vi "AlgoStim Telemetry Tool.vi"() -> ()   [LabVIEW 2010]
uses:
  Typedef Command List.ctl
  <vilib>/Instr/_visa.llb/VISA Configure Serial Port (Instr).vi
  MICS_ID Global.vi
panel:
  in  "stop":bool
  out "Busy Flag":string="ERROR"
  out "ERROR":bool
  out "SESSION":bool
  out "IDLE":bool
  out "Response":string
  in  "Tab Control":T1(tab)
  out "Error Flag":string="ERROR"
  in  "Clear Error":bool caption="Search for Device"
  out "Error Monitor":errorcluster
  in  "Query Error":bool caption="Search for Device"
  out "Base Station Errors Query":string
  in  "Dongle Reset":bool caption="Search for Device"
  in  "Base Station RF Control":T2={"CCA Mode"=FALSE, "Manual RF CH:"=2, "Base Station CCA Results"=[], "Update CCA"=FALSE, "RSSI Measurement"=0, "Use Averaging?"=TRUE, "400MHz Wakeup"=FALSE, "Listen\nfor\nEmergency"=FALSE} {"RSSI Measurement" items=["External ADC"=0, "Internal ADC"=2]; "Manual RF CH:" min=1 max=10 step=1}
  in  "Search for Device":T3 {"Detected MICS ID's" format="%06x"}
  in  "Session Control":T4={"Open Session"=FALSE, "Close Session"=FALSE, "TARGET MICS ID"=0, "EXID"=16773121, "Company ID"=187, "Calibrate Antenna on \"Open Session\"? "=TRUE} {"Company ID" format="%02x"; "EXID" format="%06x"; "TARGET MICS ID" format="%06x"}
  out "Link Status":T5={"ImplantID"=0, "CompanyID"=0, "RF_Channel"=4, "RX_Mod"=0, "TX_Mod"=0, "TXBlockSize"=15, "RXBlockSize"=15, "BlocksPerPack"=31} {"BlocksPerPack" items=["1"=1, "2"=2, "3"=3, "4"=4, "5"=5, "6"=6, "7"=7, "8"=8, "9"=9, "10"=10, "11"=11, "12"=12, "13"=13, "14"=14, "15"=15, "16"=16, "17"=17, "18"=18, "19"=19, "20"=20, "21"=21, "22"=22, "23"=23, "24"=24, "25"=25, "26"=26, "27"=27, "28"=28, "29"=29, "30"=30, "31"=31]; "RXBlockSize" items=["2"=2, "3"=3, "4"=4, "5"=5, "6"=6, "7"=7, "8"=8, "9"=9, "10"=10, "11"=11, "12"=12, "13"=13, "14"=14, "15"=15, "16"=16, "17"=17, "18"=18, "19"=19, "20"=20, "21"=21, "22"=22, "23"=23, "24"=24, "25"=25, "26"=26, "27"=27, "28"=28, "29"=29, "30"=30, "31"=31]; "TXBlockSize" items=["2"=2, "3"=3, "4"=4, "5"=5, "6"=6, "7"=7, "8"=8, "9"=9, "10"=10, "11"=11, "12"=12, "13"=13, "14"=14, "15"=15, "16"=16, "17"=17, "18"=18, "19"=19, "20"=20, "21"=21, "22"=22, "23"=23, "24"=24, "25"=25, "26"=26, "27"=27, "28"=28, "29"=29, "30"=30, "31"=31]; "TX_Mod" items=["2FSK-FB"=0, "2FSK"=2, "4FSK"=3]; "RX_Mod" items=["2FSK-FB"=0, "2FSK"=8, "4FSK"=12]; "RF_Channel" items=["0", "1", "2", "3", "4", "5", "6", "7", "8", "9"]; "CompanyID" format="%02x"; "ImplantID" format="%06x"}
  out "Link Quality":T6={"MAX_BIT_ERROR"=FALSE, "MAX_RETRIES"=FALSE, "Corrected Blocks"=2650, "CRC Errors"=2650}
  out "Data Status":T7={"TX_BlockCount"=2650, "RX_BlockCount"=2650, "DataErrorCount"=2650}
  out "Status Flags":T8
  in  "Telem Driver":bool caption="Search for Device"
  in  "Parameters":string
  out "Data":string
  out "bChecksum Valid":bool
  out "tChecksum Valid":bool
  out "Response Token":string
  out "Response Code":string
  in  "Command":T9
  in  "CP_DATA IN":u8[](array[numeric])
  out "CP_DATA OUT":u8[](array[numeric])
  in  "Get VBAT Cont":bool
  in  "Get VBAT Single":bool
  out "ADC Counts":dbl
  out "VBAT (Volts)":dbl format="%.3f"
  out "Charging Status":string
  in  "LoadPatProgSlot":u8=1 min=1 max=10 step=1
  in  "LoadPatProgFromDevice":bool caption="Search for Device"
  in  "PulsePW":u16
  in  "PulsePWDn":bool
  in  "PulsePWUp":bool
  in  "Pulse #":u8=1 min=1 max=4 step=1
  in  "PulseAmpl":u16
  in  "PulseAmpDn":bool
  in  "PulseAmpUp":bool
  in  "Freq Index":u8
  in  "ProgAmpls":u16[](array[numeric])
  in  "FreqDn":bool
  in  "FreqUp":bool
  in  "ProgAmpDn":bool
  in  "ProgAmpUp":bool
  in  "StopStimulation":bool caption="Search for Device"
  in  "StartStimulation":bool caption="Search for Device"
  in  "SetPatProgActive":bool caption="Search for Device"
  in  "SendPatProgToDevice":bool caption="Search for Device"
  in  "UpdatePatProgString":bool caption="Search for Device"
  in  "Patient Program String":string
  in  "ResetPatProgToDefaults":bool caption="Search for Device"
  in  "LoadPatProgFromFile":bool caption="Search for Device"
  in  "SavePatProgToFile":bool caption="Search for Device"
  in  "PatStim":T10={"PA"={"Defined"=FALSE, "Amplitudes"=[0, 0, 0, 0, 0, 0, 0, 0, 0, 0, 0, 0, 0, 0, 0, 0, 0, 0, 0, 0, 0, 0, 0, 0, 0, 0], "Pulse Name"="", "Label.Ch"=["ch1", "ch2", "ch3", "ch4", "ch5", "ch6", "ch7", "ch8", "ch9", "ch10", "ch11", "ch12", "ch13", "ch14", "ch15", "ch16", "ch17", "ch18", "ch19", "ch20", "ch21", "ch22", "ch23", "ch24", "ch25", "ch26"], "Amp Low Limit (uA)"=0, "Amp Step (uA)"=0, "Amp Step Index"=0, "PW Low Limit (uS)"=0, "PW High Limit (uS)"=0, "PW Default (uS)"=0}, "Allowed Freq Indexes"=[], "PB"={"Defined"=FALSE, "Amplitudes"=[0, 0, 0, 0, 0, 0, 0, 0, 0, 0, 0, 0, 0, 0, 0, 0, 0, 0, 0, 0, 0, 0, 0, 0, 0, 0], "Pulse Name"="", "Label.Ch"=["ch1", "ch2", "ch3", "ch4", "ch5", "ch6", "ch7", "ch8", "ch9", "ch10", "ch11", "ch12", "ch13", "ch14", "ch15", "ch16", "ch17", "ch18", "ch19", "ch20", "ch21", "ch22", "ch23", "ch24", "ch25", "ch26"], "Amp Low Limit (uA)"=0, "Amp Step (uA)"=0, "Amp Step Index"=0, "PW Low Limit (uS)"=0, "PW High Limit (uS)"=0, "PW Default (uS)"=0}, "PC"={"Defined"=FALSE, "Amplitudes"=[0, 0, 0, 0, 0, 0, 0, 0, 0, 0, 0, 0, 0, 0, 0, 0, 0, 0, 0, 0, 0, 0, 0, 0, 0, 0], "Pulse Name"="", "Label.Ch"=["ch1", "ch2", "ch3", "ch4", "ch5", "ch6", "ch7", "ch8", "ch9", "ch10", "ch11", "ch12", "ch13", "ch14", "ch15", "ch16", "ch17", "ch18", "ch19", "ch20", "ch21", "ch22", "ch23", "ch24", "ch25", "ch26"], "Amp Low Limit (uA)"=0, "Amp Step (uA)"=0, "Amp Step Index"=0, "PW Low Limit (uS)"=0, "PW High Limit (uS)"=0, "PW Default (uS)"=0}, "PD"={"Defined"=FALSE, "Amplitudes"=[0, 0, 0, 0, 0, 0, 0, 0, 0, 0, 0, 0, 0, 0, 0, 0, 0, 0, 0, 0, 0, 0, 0, 0, 0, 0], "Pulse Name"="", "Label.Ch"=["ch1", "ch2", "ch3", "ch4", "ch5", "ch6", "ch7", "ch8", "ch9", "ch10", "ch11", "ch12", "ch13", "ch14", "ch15", "ch16", "ch17", "ch18", "ch19", "ch20", "ch21", "ch22", "ch23", "ch24", "ch25", "ch26"], "Amp Low Limit (uA)"=0, "Amp Step (uA)"=0, "Amp Step Index"=0, "PW Low Limit (uS)"=0, "PW High Limit (uS)"=0, "PW Default (uS)"=0}, "label.freqindex"=[], "Default Freq Index"=0, "Program Name"="", "Program Number"=0, "Program Defined"=FALSE, "Program Disabled"=FALSE} {"Allowed Freq Indexes" format="%02x"}
  in  "Set Attenuator":bool caption="Search for Device"
  in  "Get Attenuator":bool caption="Search for Device"
  in  "Attenuation (dB)":dbl min=0.0 max=31.75 step=0.25 format="%.2g"
  in  "File Path":path
  in  "ZL Mass Read":bool caption="Search for Device"
  out "Get Data Dec":u8
  in  "Register":u16(ring)=1000 items=["---MANUAL ENTRY---"=1000, "REG_NOREG"=0, "REG_RXBUFF_USED"=1, "REG_RXBUFF_BSIZE"=2, "REG_TXBUFF_USED"=3, "REG_TXBUFF_BSIZE"=4, "REG_TXBUFF_MAXPACKSIZE"=5, "REG_MAC_ERRCLR"=6, "REG_MAC_TRAINNUM"=7, "REG_MAC_SYNCMATCH"=8, "REG_MAC_SYNC1"=9, "REG_MAC_SYNC2"=10, "REG_MAC_SYNC3"=11, "REG_MAC_SYNC4"=12, "REG_MAC_SYNC5"=13, "REG_MAC_MAXBERR"=14, "REG_MAC_ECCORR"=15, "REG_MAC_CRCERR"=16, "REG_MAC_BLKCNT1"=17, "REG_MAC_BLKCNT2"=18, "REG_MAC_IMDTRANSID1"=19, "REG_MAC_IMDTRANSID2"=20, "REG_MAC_IMDTRANSID3"=21, "REG_MAC_COMPANYID"=22, "REG_MAC_MODUSER"=23, "REG_MAC_CHANNEL"=25, "REG_MAC_CLEARWDOG"=26, "REG_MAC_CKCORRTHRESH"=27, "REG_HK_TXADDR"=28, "REG_HK_TXDATA"=29, "REG_HK_TXREPLY"=30, "REG_HK_USERDATA"=31, "REG_HK_USERSTATUS"=32, "REG_HK_LASTADDRESS"=33, "REG_HK_MODE"=34, "REG_MAC_STATUSSEQ"=35, "REG_MAC_MAXRETRIES"=36, "REG_MAC_RESENDTIME"=37, "REG_MAC_POWERSAVETIME"=38, "REG_MAC_HEAD_DET"=39, "REG_MAC_CTRL"=41, "REG_MAC_INITCOM"=42, "REG_INTERFACE_MODE"=43, "REG_TXRXBUFF_BOTH"=44, "REG_TXRXBUFF"=45, "REG_IRQ_RAWSTATUS1"=46, "REG_IRQ_ENABLE1"=47, "REG_IRQ_ENABLESET1"=48, "REG_IRQ_ENABLECLEAR1"=49, "REG_IRQ_RAWSTATUS2"=50, "REG_IRQ_ENABLE2"=51, "REG_IRQ_ENABLESET2"=52, "REG_IRQ_ENABLECLEAR2"=53, "REG_IRQ_STATUS1"=54, "REG_IRQ_STATUS2"=55, "REG_IRQ_AUXSTATUS"=56, "REG_TXBUFF_OVERFLOW"=57, "REG_PO0"=58, "REG_P01"=59, "REG_P02"=60, "REG_P03"=61, "REG_GP0"=62, "REG_GPI"=63, "REG_WAKEUP_245IN"=64, "REG_WAKEUP_COMPANYID"=65, "REG_WAKEUP_IMDTRANSID1"=66, "REG_WAKEUP_IMDTRANSID2"=67, "REG_WAKEUP_IMDTRANSID3"=68, "REG_WAKEUP_CHANNEL"=69, "REG_WAKEUP_MODUSER"=70, "REG_WAKEUP_DEVICEMODE"=71, "REG_WAKEUP_WK_RX_CTRL1"=72, "REG_WAKEUP_STACK_ADDR"=73, "REG_WAKEUP_CTRL"=74, "REG_WAKEUP_STROSCRTRIM"=75, "REG_WAKEUP_BIASTRIM"=76, "REG_WAKEUP_ANT245TUNE"=77, "REG_WAKEUP_WK_RX_RTRIMDET"=78, "REG_WAKEUP_WK_RX_RTRIMDEMOD"=79, "REG_WAKEUP_WK_RX_RSSIGAIN"=80, "REG_WAKEUP_LNAFREQ1"=81, "REG_WAKEUP_STACK"=83, "REG_WAKUP_XOSU"=84, "REG_WAKUP_CNTDROPOUT"=85, "REG_WAKEUP_CRCCTRL"=86, "REG_WAKEUP_CRCWORD1"=87, "REG_WAKEUP_CRCWORD2"=88, "REG_WAKEUP_WK_RX_CTRIM"=89, "REG_WAKEUP_VDDATRIM"=90, "REG_WAKEUP_VDDDTRIM"=91, "REG_WAKEUP_TESTIOBUFEN"=92, "REG_WAKEUP_TESTIOCLAMP"=93, "CORE_RESET_ADDRESS"=94, "CHIP_RESET_ADDRESS"=95, "REG_RF_TXGENCTRL"=96, "REG_RF_TXIFCTRL"=97, "REG_RF_TXRF_SEL_CTRL"=98, "REG_RF_TXRFPWRDEFAULTSET"=99, "REG_RF_RSSITRIM"=100, "REG_RF_TXIFOSCTUNE"=101, "REG_RF_TXIFGAINIMB"=102, "REG_RF_TXIFLOCK"=103, "REG_RF_RXRFLNAGAINTRIM"=104, "REG_RF_RXBIASTR"=105, "REG_RF_RXGENCTRL"=106, "REG_RF_RXIFADCDECLEV"=107, "REG_RF_RXIFDETFILTERTUNE"=108, "REG_RF_RXIFFILTERTUNE"=109, "REG_RF_GENENABLES"=110, "REG_RF_SYNTH_CHANNEL"=111, "REG_TX_RAMP_RTRIM"=112, "REG_TX_RAMP_CTRIM"=113, "REG_RF_XO_TRIM"=114, "REG_RF_SYNTH_SET_TRIM"=115, "REG_RF_ADCCTRL"=116, "REG_RF_ADCOUTPUT"=117, "REG_RF_TXIFAMP"=118, "REG_RF_SYNTH_RTRIM"=119, "REG_RF_SYNTH_CTRIM"=120, "REG_RF_SYNTH_CT"=121, "REG_RF_TXMIXER_IOSTRIM_HIGH_IP"=122, "REG_RF_TXMIXER_IOSTRIM_HIGH_IN"=123, "REG_RF_TXMIXER_IOSTRIM_HIGH_QP"=124, "REG_RF_TXMIXER_IOSTRIM_HIGH_QN"=125, "REG_HX_WUADDR"=126, "REG_REVISION"=127, "REG_NOREG_TEST"=128, "REG_DTEST_RXBUFF"=129, "REG_RXBUFF_NEXT_BLOCK"=130, "REG_RXBUFF_FIRST_IN_PACK"=131, "REG_RXBUFF_FIRST_EMPTY"=132, "REG_MAC_BYPASS"=133, "REG_DTEST_TXBUFF"=134, "REG_TXBUFF_NEXT_BLOCK"=135, "REG_TXBUFF_FIRST_IN_PACK"=136, "REG_TXBUFF_FIRST_EMPTY"=137, "REG_DTEST_SEQ"=138, "REG_DTEST_CKCORR"=139, "REG_MAC_TOPSTATE"=140, "REG_DTEST_INTERFACE"=141, "REG_IFACE_TXRX_BYPASS"=142, "REG_MAC_TXRXWAIT"=143, "REG_MAC_TXRFRAMP"=144, "REG_MAC_TRAINWORD"=145, "REG_MAC_TRAINWORD2"=146, "REG_MAC_SETTINGS"=147, "REG_MAC_CALSELECT1"=148, "REG_MAC_CALSELECT2"=149, "REG_MAC_ANTMATCHSEL"=150, "REG_MAC_ANTTUNESEL1"=151, "REG_MAC_ANTTUNESEL2"=152, "REG_MAC_ANTTUNESEL3"=153, "REG_MAC_ANTTUNESTEP"=154, "REG_MAC_WUMODEBURST"=156, "REG_MAC_WUOFFSHORT"=157, "REG_MAC_WUOFFLONG"=158, "REG_MAC_CLKRECCTRL"=159, "REG_HK_MODE_P2"=162, "REG_MAC_ANTTUNERES1"=164, "REG_MAC_ANTTUNERES2"=165, "REG_INTERFACE_MODE_TEST"=171, "REG_TXRXBUFF_BOTH_P2"=172, "REG_TXRXBUFF_P2"=173, "REG_IRQ_RAWSTATUS1_P2"=174, "REG_MAC_TXIFSTATUS1"=176, "REG_MAC_TXIFSTATUS2"=177, "REG_IRQ_RAWSTATUS2_P2"=178, "REG_MAC_TXIFRAMPDELAY"=179, "REG_MAC_TXIFRAMPSLOPE"=180, "REG_MAX_TXIFRAMP"=181, "REG_IRQ_STATUS1_P2"=182, "REG_IRQ_STATUS2_P2"=183, "REG_IRQ_AUXSTATUS_P2"=184, "REG_MAC_UNLOCK"=188, "REG_MAC_TXIFFREQ"=190, "REG_WAKEUP_TESTCTRL1"=192, "REG_WAKEUP_RX_EN_CNT"=193, "REG_WAKEUP_TESTENABLES"=194, "REG_WAKEUP_DTBI_CTRL"=195, "REG_WAKEUP_DTBO_CTRL"=196, "REG_WAKEUP_TESTIOBUFTEST"=197, "REG_WAKEUP_WK_RX_TESTCTRL1"=198, "REG_WAKEUP_WK_RX_TESTCTRL2"=199, "REG_WAKEUP_SENS_SEQUENCE_CTRL"=200, "REG_WAKEUP_LNABIAS"=201, "REG_WAKEUP_DET_TH_TRIM1"=202, "REG_WAKEUP_LNABIAS_NOM1"=203, "REG_WAKEUP_RX_TSHORT_TRIM1"=204, "REG_WAKEUP_LNABIAS_NOM2"=205, "REG_WAKEUP_RX_TLONG_TRIM1"=206, "REG_WAKEUP_LNA_NEGRTRIM_NOM1"=207, "REG_WAKEUP_RX_TBURST_TRIM1"=208, "REG_WAKEUP_RX_LNA_NEGRTRIM_NOM2"=209, "REG_WAKEUP_RX_BB_G_BW_SEL1"=210, "REG_WAKEUP_WK_RX_DET_IOSTRIM1"=212, "REG_WAKEUP_WK_RX_CTRL2"=214, "REG_WAKEUP_WK_RX_RSSIVOSTRIM"=215, "REG_WAKEUP_LNANEGR_EFF"=216, "REG_WAKEUP_XOSU_FAST"=217, "REG_WAKEUP_STROSCPWIDTH1"=218, "REG_WAKEUP_STROSCPERIOD1"=220, "REG_WAKEUP_STROSCPERIOD2"=221, "REG_WAKEUP_WK_RX_LNA_NEGRTRIM1"=222, "REG_RF_TXTESTENABLE"=224, "REG_RF_TXIFTESTMODE"=225, "REG_RF_RXTESTENABLE"=226, "REG_RF_RXIFTESTCTRL1"=227, "REG_RF_RXIFTESTCTRL2"=228, "REG_RF_RXIFTESTCTRL3"=229, "REG_RF_SYNTH_TESTCTRL1"=230, "REG_RF_SYNTH_TESTCTRL2"=231, "REG_RF_SYNTH_TESTCTRL3"=232, "REG_RF_ADCTEST1"=237, "REG_RF_ADCTEST2"=238, "REG_RF_TXMIXER_IOSTRIM_LOW_IP"=240, "REG_RF_TXMIXER_IOSTRIM_LOW_IN"=241, "REG_RF_TXMIXER_ISOTRIM_LOW_QP"=242, "REG_RF_TXMIXER_IOSTRIM_LOW_QN"=243, "REG_RF_SYNTH_KPD"=244, "REG_RF_SYNTH_LOLEV"=245, "REG_RF_TXRFPWRTUNEANTSET"=246, "REG_RF_TXPD_GAIN_CTRL"=247, "REG_RF_SYNTH_STARTUP"=248, "REG_RF_TXRFANTTUNE_TXMODE"=249, "REG_RF_TXRFANTTUNE_RXMODE"=250, "REG_RF_RXRFANTTUNE_TXMODE"=251, "REG_RF_RXRFANTTUNE_RXMODE"=252, "REG_ANTMATCH1"=253, "REG_ANTMATCH2"=254, "REG_REVISION_P2"=255]
  in  "Set Register":bool caption="Search for Device"
  in  "Get Register":bool caption="Search for Device"
  in  "Use Remote?":bool
  out "Get Data":u8 format="%02x"
  in  "Set Data":u8 format="%02x"
  in  "Address":u16 format="%04x"
  in  "Do Calibration":bool caption="Search for Device"
  in  "CAL_WAKEUP_STROBE_OSC":bool
  in  "MICS Channel":i8
  in  "Execute on Remote?(F)":bool
  in  "CAL_TX_IF_OSC":bool
  in  "CAL_FM_DETECT_AND_RX_IF":bool
  in  "CAL_RX_ADC":bool
  in  "CAL_400_MHZ_TX":bool
  in  "CAL_400_MHZ_RX":bool
  in  "CAL_400_MHZ_ANT":bool
  in  "CAL_24MHZ_CRYSTAL_OSC":bool
  in  "Tick Count":u32
  out "error out":errorcluster
  in  "error in (no error)":errorcluster
  in  "VISA Resource Name":refnum<visa-resource-name>="COM14"
  in  "Default MICS Config":T11={"ConfigFlags"=0, "ImplantID"=1048576, "CompanyID"=187, "Normal_Comm"={"RF_Channel"=4, "UserData"=0, "TX_Mod"=0, "RX_Mod"=0, "RX_BlockSize"=15, "BlockPerPack"=31, "TX_BlockSize"=15}, "Emerg_Comm"={"RF_Channel"=4, "UserData"=0, "TX_Mod"=0, "RX_Mod"=0, "TX_BlockSize"=15, "BlockPerPack"=31, "RX_BlockSize"=15}, "ImplantRev"=4, "245TX_PowerCal"=0, "245TX_Power"=10, "CCA_RSSI_Thresholds"={"ch0"=2650, "ch1"=2650, "ch2"=2650, "ch3"=2650, "ch4"=2650, "ch5"=2650, "ch6"=2650, "ch7"=2650, "ch8"=2650, "ch9"=2650}} {"ImplantID" format="%x"; "Normal_Comm"."RF_Channel" items=["0", "1", "2", "3", "4", "5", "6", "7", "8", "9"]; "Normal_Comm"."UserData" items=["0 - 000"=0, "1 - 001"=16, "2 - 010"=32, "3 - 011"=48, "4 - 100"=64, "5 - 101"=80, "6 - 110"=96, "7 - 111"=112]; "Normal_Comm"."TX_Mod" items=["2FSK-FB"=0, "2FSK"=2, "4FSK"=3]; "Normal_Comm"."RX_Mod" items=["2FSK-FB"=0, "2FSK"=8, "4FSK"=12]; "Normal_Comm"."RX_BlockSize" items=["2"=2, "3"=3, "4"=4, "5"=5, "6"=6, "7"=7, "8"=8, "9"=9, "10"=10, "11"=11, "12"=12, "13"=13, "14"=14, "15"=15, "16"=16, "17"=17, "18"=18, "19"=19, "20"=20, "21"=21, "22"=22, "23"=23, "24"=24, "25"=25, "26"=26, "27"=27, "28"=28, "29"=29, "30"=30, "31"=31]; "Normal_Comm"."BlockPerPack" items=["1"=1, "2"=2, "3"=3, "4"=4, "5"=5, "6"=6, "7"=7, "8"=8, "9"=9, "10"=10, "11"=11, "12"=12, "13"=13, "14"=14, "15"=15, "16"=16, "17"=17, "18"=18, "19"=19, "20"=20, "21"=21, "22"=22, "23"=23, "24"=24, "25"=25, "26"=26, "27"=27, "28"=28, "29"=29, "30"=30, "31"=31]; "Normal_Comm"."TX_BlockSize" items=["2"=2, "3"=3, "4"=4, "5"=5, "6"=6, "7"=7, "8"=8, "9"=9, "10"=10, "11"=11, "12"=12, "13"=13, "14"=14, "15"=15, "16"=16, "17"=17, "18"=18, "19"=19, "20"=20, "21"=21, "22"=22, "23"=23, "24"=24, "25"=25, "26"=26, "27"=27, "28"=28, "29"=29, "30"=30, "31"=31]; "Emerg_Comm"."RF_Channel" items=["0", "1", "2", "3", "4", "5", "6", "7", "8", "9"]; "Emerg_Comm"."UserData" items=["0 - 000"=0, "1 - 001"=16, "2 - 010"=32, "3 - 011"=48, "4 - 100"=64, "5 - 101"=80, "6 - 110"=96, "7 - 111"=112]; "Emerg_Comm"."TX_Mod" items=["2FSK-FB"=0, "2FSK"=2, "4FSK"=3]; "Emerg_Comm"."RX_Mod" items=["2FSK-FB"=0, "2FSK"=8, "4FSK"=12]; "Emerg_Comm"."TX_BlockSize" items=["2"=2, "3"=3, "4"=4, "5"=5, "6"=6, "7"=7, "8"=8, "9"=9, "10"=10, "11"=11, "12"=12, "13"=13, "14"=14, "15"=15, "16"=16, "17"=17, "18"=18, "19"=19, "20"=20, "21"=21, "22"=22, "23"=23, "24"=24, "25"=25, "26"=26, "27"=27, "28"=28, "29"=29, "30"=30, "31"=31]; "Emerg_Comm"."BlockPerPack" items=["1"=1, "2"=2, "3"=3, "4"=4, "5"=5, "6"=6, "7"=7, "8"=8, "9"=9, "10"=10, "11"=11, "12"=12, "13"=13, "14"=14, "15"=15, "16"=16, "17"=17, "18"=18, "19"=19, "20"=20, "21"=21, "22"=22, "23"=23, "24"=24, "25"=25, "26"=26, "27"=27, "28"=28, "29"=29, "30"=30, "31"=31]; "Emerg_Comm"."RX_BlockSize" items=["2"=2, "3"=3, "4"=4, "5"=5, "6"=6, "7"=7, "8"=8, "9"=9, "10"=10, "11"=11, "12"=12, "13"=13, "14"=14, "15"=15, "16"=16, "17"=17, "18"=18, "19"=19, "20"=20, "21"=21, "22"=22, "23"=23, "24"=24, "25"=25, "26"=26, "27"=27, "28"=28, "29"=29, "30"=30, "31"=31]; "ImplantRev" items=["ZL70100"=0, "ZL70101"=1, "ZL70102"=4]; "245TX_PowerCal" items=["-29"=-29, "-4"=-4, "-2"=-2, "0"=0, "2"=2, "4"=4, "6"=6, "8"=8, "10"=10, "12"=12, "14"=14, "16"=16, "18"=18, "20"=20, "22"=22, "24"=24, "26"=26, "27"=27]; "245TX_Power" items=["-29"=-29, "-4"=-4, "-2"=-2, "0"=0, "2"=2, "4"=4, "6"=6, "8"=8, "10"=10, "12"=12, "14"=14, "16"=16, "18"=18, "20"=20, "22"=22, "24"=24, "26"=26, "27"=27]}
  # "400MHz\nWakeup"
  # "Auto CCA"
  # "Battery State of Charge"
  # "x .001205 ="
  # "Program Adjust"
  # "Pulse Adjust"
  # "PA"
  # "PB"
  # "PC"
  # "PD"
  # "Pulse D"
  # "Pulse C"
  # "Pulse B"
  # "Pulse A"
  # "ZL REGISTER PEEK AND POKE"
  # "ZL REGISTER MASS READ TO FILE"
  # "Use \"Register\" menu list for named registers,\nor leave it on \"Manual Entry\" and use the \n\"Address\" control to select a register address.\n          (Add 128 (0x80) to P2 addresses)"
  # "Use this function to copy all Zarlink registers to\na text file."
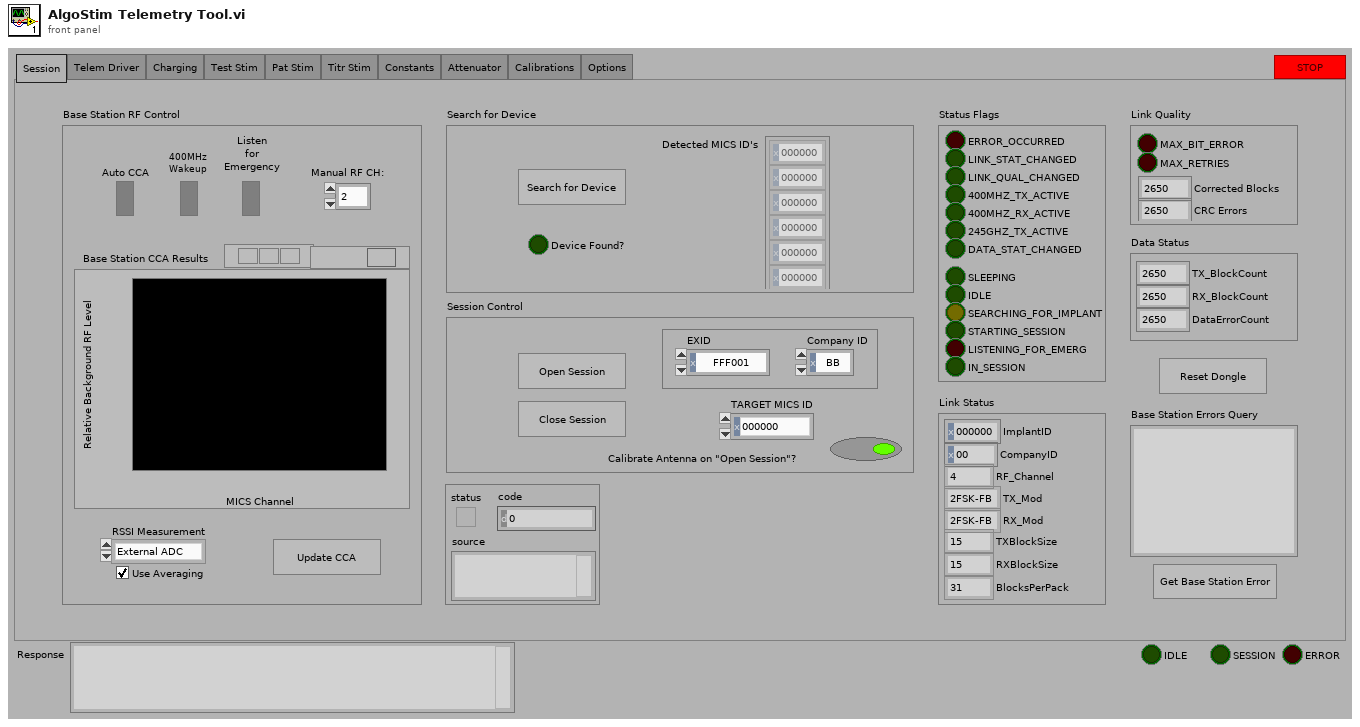
[diagram p1: front panel]
types:
  T1 = enum32{"Session", "Telem Driver", "Charging", "Test Stim", "Pat Stim", "Titr Stim", "Constants", "Attenuator", "Calibrations", "Options"}
  T2 = cluster{"CCA Mode":bool, "Manual RF CH:":u8, "Base Station CCA Results":dbl[], "Update CCA":bool, "RSSI Measurement":u16, "Use Averaging?":bool, "400MHz Wakeup":bool, "Listen\nfor\nEmergency":bool}
  T3 = cluster{"Search for Device":bool, "Device Found?":bool, "Detected MICS ID's":u32[]}
  T4 = cluster{"Open Session":bool, "Close Session":bool, "TARGET MICS ID":u32, "EXID":u32, "Company ID":u8, "Calibrate Antenna on \"Open Session\"? ":bool}
  T5 = cluster{"ImplantID":u32, "CompanyID":u8, "RF_Channel":u8, "RX_Mod":u8, "TX_Mod":u8, "TXBlockSize":u8, "RXBlockSize":u8, "BlocksPerPack":u8}
  T6 = cluster{"MAX_BIT_ERROR":bool, "MAX_RETRIES":bool, "Corrected Blocks":u16, "CRC Errors":u16}
  T7 = cluster{"TX_BlockCount":u16, "RX_BlockCount":u16, "DataErrorCount":u16}
  T8 = cluster{"ERROR_OCCURRED":bool, "LINK_STAT_CHANGED":bool, "LINK_QUAL_CHANGED":bool, "400MHZ_TX_ACTIVE":bool, "400MHZ_RX_ACTIVE":bool, "245GHZ_TX_ACTIVE":bool, "DATA_STAT_CHANGED":bool, "SLEEPING":bool, "IDLE":bool, "SEARCHING_FOR_IMPLANT":bool, "STARTING_SESSION":bool, "LISTENING_FOR_EMERG":bool, "IN_SESSION":bool}
  T9 = typedef "Typedef Command List.ctl" = enum16{"Get xPG Status", "xPG Stimulation", "Select Program", "Increment Program Amplitude", "Decrement Program Amplitude", "Get PoP Constants", "Get PPC Constants", "Get Program Names", "Set Pulse Amplitude", "Increment Pulse Amplitude", "Decrement Pulse Amplitude", "Get Pulse Widths", "Set Pulse Widths", "Increment Pulse Width", "Decrement Pulse Width", "Get Program Frequency", "Set Program Frequency", "Increment Program Frequency", "Decrement Program Frequency", "Inject Event", "Charging Control", "Get xPG Identity", "Set xPG Identity", "Restore Program Defaults", "Get Program Definition", "Set Program Definition", "Get Program Constants", "Set Program Constants", "Get Configurable Device Parameters", "Set Configurable Device Parameters", "Get Pulse Constants", "Set Pulse Constants", "Get Lead Limits", "Set Lead Limits", "Get Channel Calibrations", "Set Channel Calibrations", "<reserved 2>", "<reserved 3>", "<reserved 4>", "<reserved 5>", "<reserved 6>", "<reserved 7>", "Get Stim Asic HV Calibrations", "Set Stim Asic HV Calibrations", "<reserved 8>", "<reserved 9>", "Get CP Data", "Set CP Data", "Clear Log", "Read Log", "Append Log", "Get Patient Program Runtime", "Set Patient Program Runtime", "Impedance Measurement", "Enter Storage Mode", "Echo Short", "Echo Long", "Get General Calibration", "Set General Calibration", "Get Trim List", "Set Trim List", "Get Counter", "Set Counter", "Get Test Stimulation", "Set Test Stimulation", "Get Titration Stimulation", "Set Titration Stimulation", "Get Ramp Time", "Set Ramp Time", "Get VBAT", "Set Software Description Block", "Get Software Description Block", "Write Memory", "Read Memory", "Reset xPG", "Erase Flash Block", "Write Vectors", "Read Vectors", "Diagnostic Data", "Set Background Impedance", "Get Background Impedence ", "Set Test Waveform", "Calibrate Channel", "Get Log Range", "Reserved 0x55", "Reserved 0x56", "MICS Options", "Pair PPC", "Pair POP", "Stop Bootloader", "Tune MICS", "MICS Diagnostics", "Undefined"}
  T10 = cluster{"PA":cluster{"Defined":bool, "Amplitudes":i8[], "Pulse Name":string, "Label.Ch":string[], "Amp Low Limit (uA)":u16, "Amp Step (uA)":u16, "Amp Step Index":u16, "PW Low Limit (uS)":u16, "PW High Limit (uS)":u16, "PW Default (uS)":u16}, "Allowed Freq Indexes":u8[], "PB":cluster{"Defined":bool, "Amplitudes":i8[], "Pulse Name":string, "Label.Ch":string[], "Amp Low Limit (uA)":u16, "Amp Step (uA)":u16, "Amp Step Index":u16, "PW Low Limit (uS)":u16, "PW High Limit (uS)":u16, "PW Default (uS)":u16}, "PC":cluster{"Defined":bool, "Amplitudes":i8[], "Pulse Name":string, "Label.Ch":string[], "Amp Low Limit (uA)":u16, "Amp Step (uA)":u16, "Amp Step Index":u16, "PW Low Limit (uS)":u16, "PW High Limit (uS)":u16, "PW Default (uS)":u16}, "PD":cluster{"Defined":bool, "Amplitudes":i8[], "Pulse Name":string, "Label.Ch":string[], "Amp Low Limit (uA)":u16, "Amp Step (uA)":u16, "Amp Step Index":u16, "PW Low Limit (uS)":u16, "PW High Limit (uS)":u16, "PW Default (uS)":u16}, "label.freqindex":string[], "Default Freq Index":u8, "Program Name":string, "Program Number":u8, "Program Defined":bool, "Program Disabled":bool}
  T11 = cluster{"ConfigFlags":u8, "ImplantID":u32, "CompanyID":u8, "Normal_Comm":cluster{"RF_Channel":u8, "UserData":u8, "TX_Mod":u8, "RX_Mod":u8, "RX_BlockSize":u8, "BlockPerPack":u8, "TX_BlockSize":u8}, "Emerg_Comm":cluster{"RF_Channel":u8, "UserData":u8, "TX_Mod":u8, "RX_Mod":u8, "TX_BlockSize":u8, "BlockPerPack":u8, "RX_BlockSize":u8}, "ImplantRev":u8, "245TX_PowerCal":i8, "245TX_Power":i8, "CCA_RSSI_Thresholds":cluster{"ch0":u16, "ch1":u16, "ch2":u16, "ch3":u16, "ch4":u16, "ch5":u16, "ch6":u16, "ch7":u16, "ch8":u16, "ch9":u16}}
  T12 = cluster{"Command":T9, "Function":enum16{"Open Session", "Close Session", "Downlink Only", "Uplink Only", "Transceive (DN -> UP)"}, "MICS_ID":u32, "EXID":u32, "Use Local":bool, "Transceive Delay mS":dbl, "CP_DATA IN":u8[], "Parameters":string}
  T13 = enum16{"Open Session", "Close Session", "Downlink Only", "Uplink Only", "Transceive (DN -> UP)"}
  T14 = enum16{"Get Device Type", "Get Device Name", "Get Device Version", "Get Device Error"}
  T15 = enum16{"open", "replace", "create", "open or create", "replace or create", "replace or create with confirmation"}
  T16 = cluster{"Response Token":string, "Response Code":string, "bChecksum Valid":bool, "tChecksum Valid":bool, "CP_DATA OUT":u8[], "Data":string}
  T17 = cluster{"Open Session":bool, "Close Session":bool, "TARGET MICS ID":u32, "EXID":u32, "Company ID":u8, bool}
  T18 = cluster{"Allowed Freq Indexes[0]":u8, "Allowed Freq Indexes[1]":u8, "Allowed Freq Indexes[2]":u8, "Allowed Freq Indexes[3]":u8, "Allowed Freq Indexes[4]":u8, "Allowed Freq Indexes[5]":u8, "Allowed Freq Indexes[6]":u8, "Allowed Freq Indexes[7]":u8}
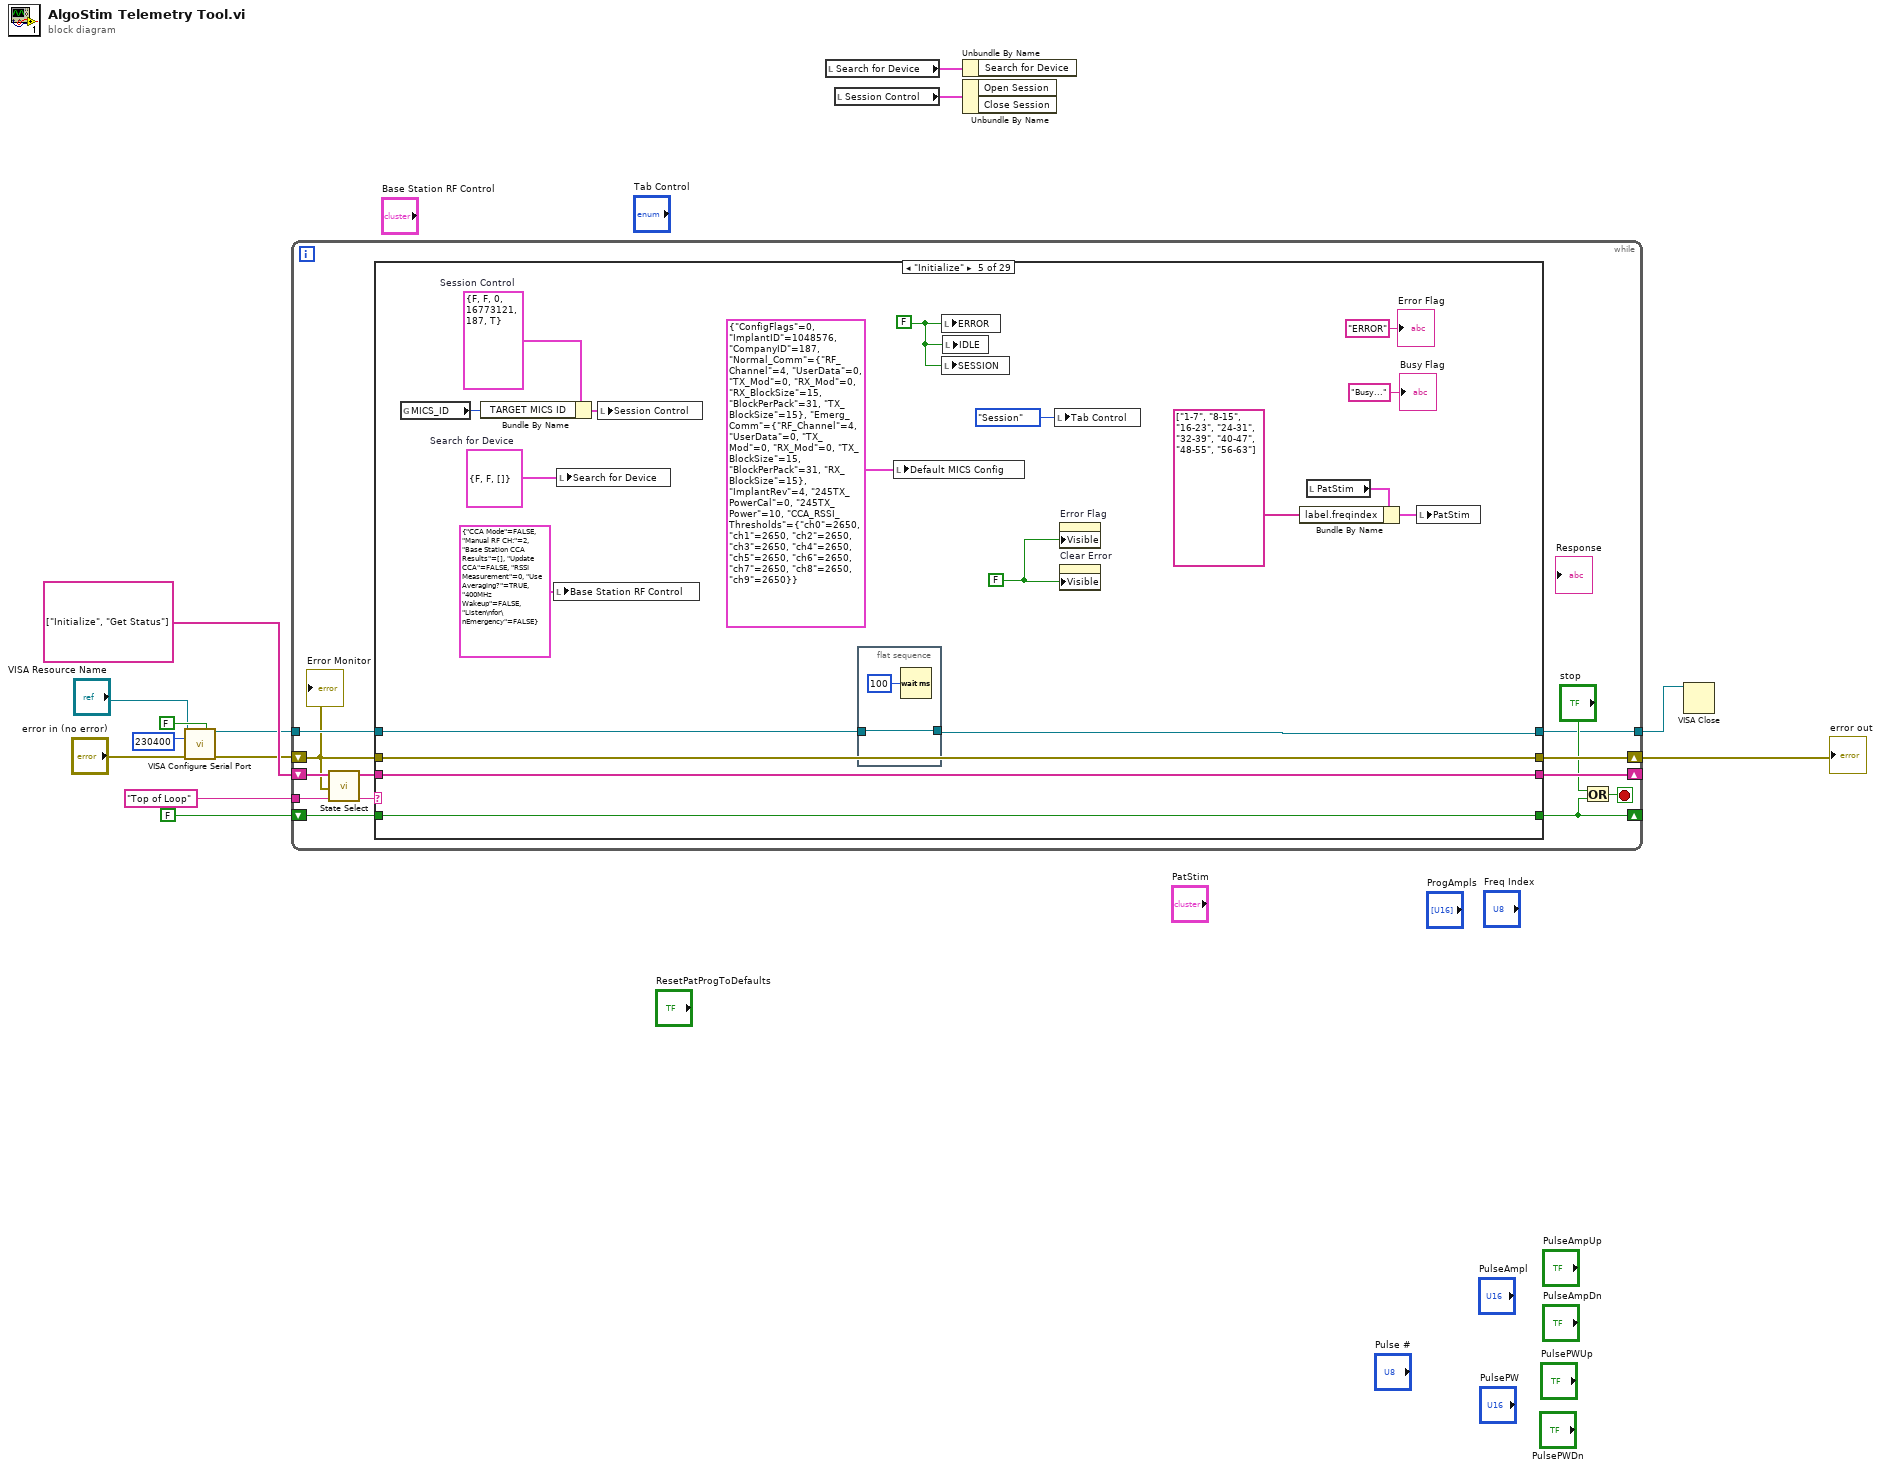
[diagram p0: block diagram]
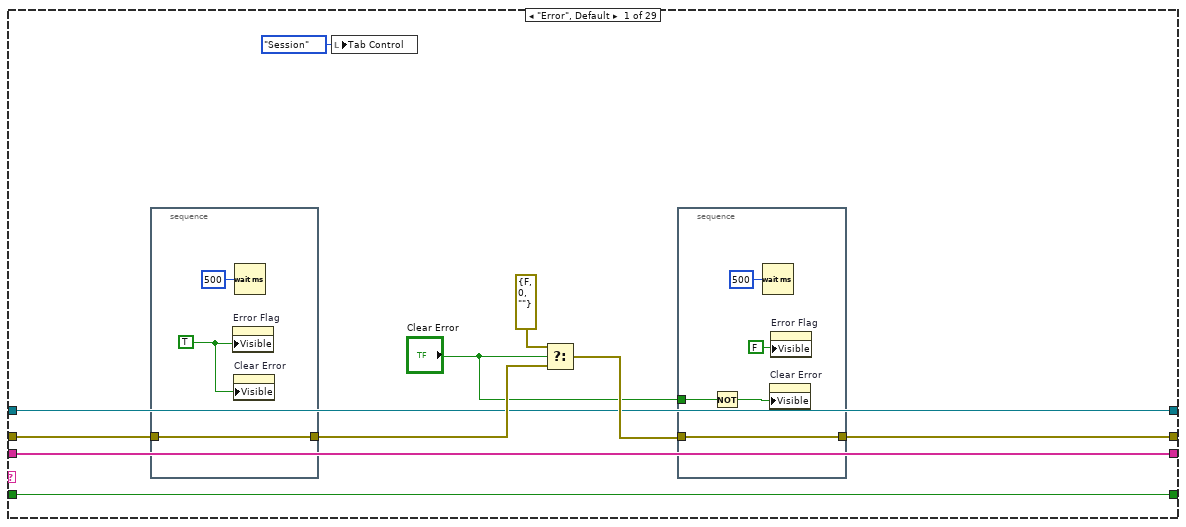
[diagram p2: hidden frame]
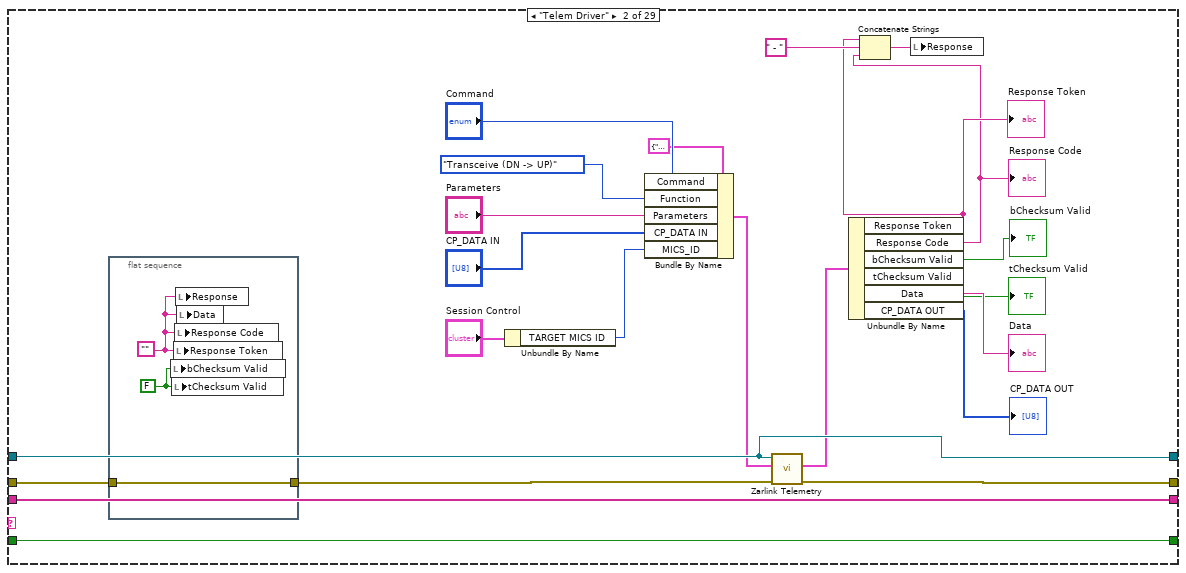
[diagram p3: hidden frame]
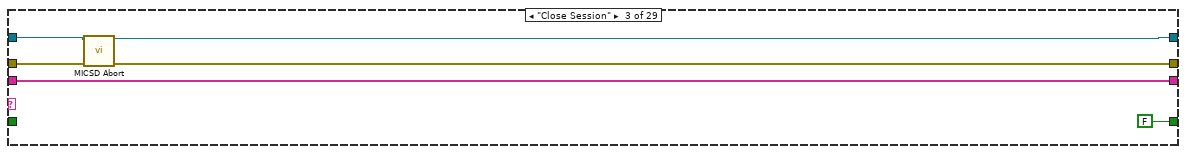
[diagram p4: hidden frame]
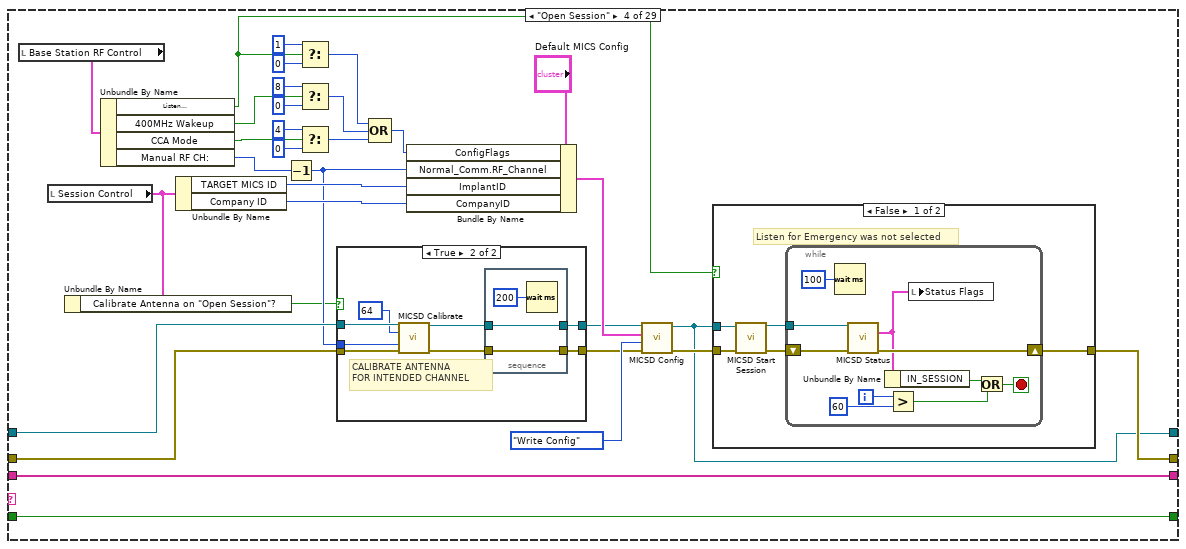
[diagram p5: hidden frame]
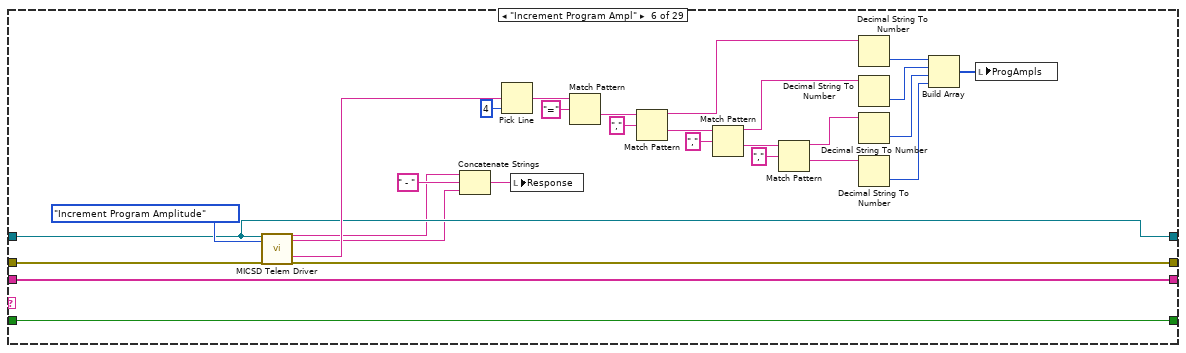
[diagram p8: hidden frame]
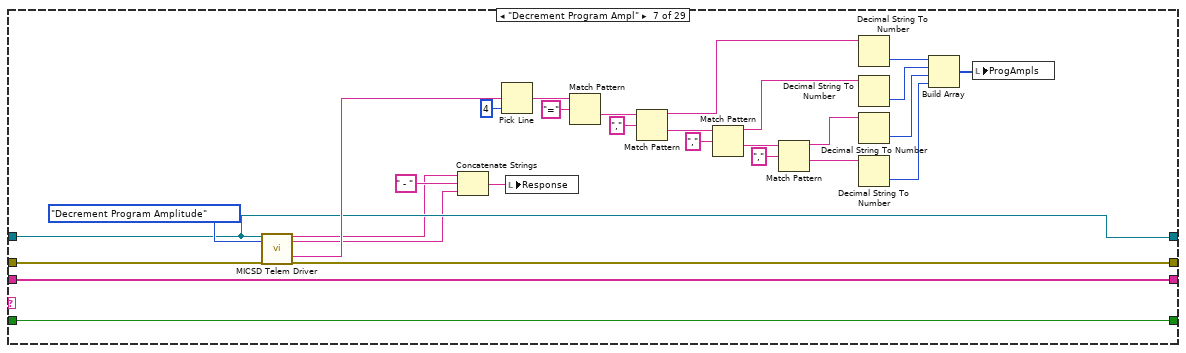
[diagram p9: hidden frame]
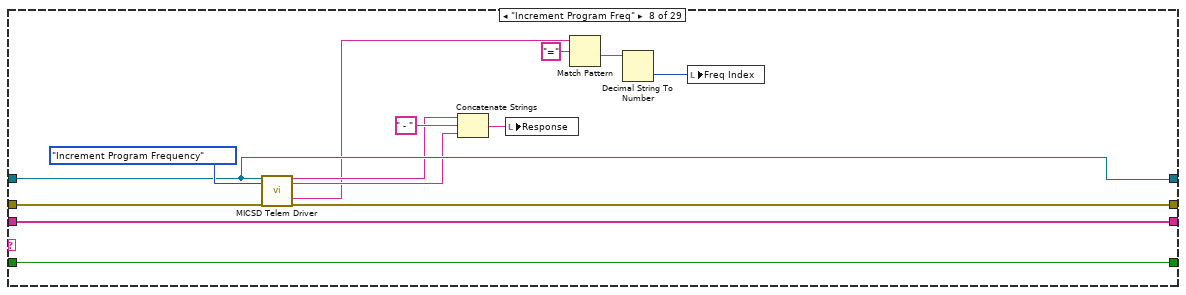
[diagram p10: hidden frame]
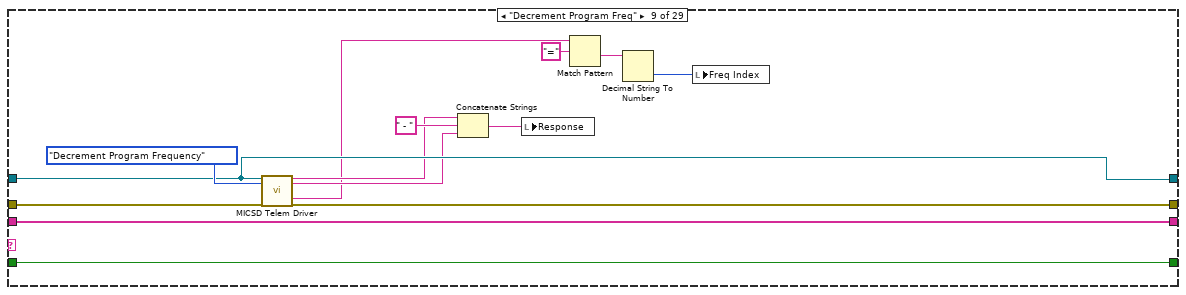
[diagram p11: hidden frame]
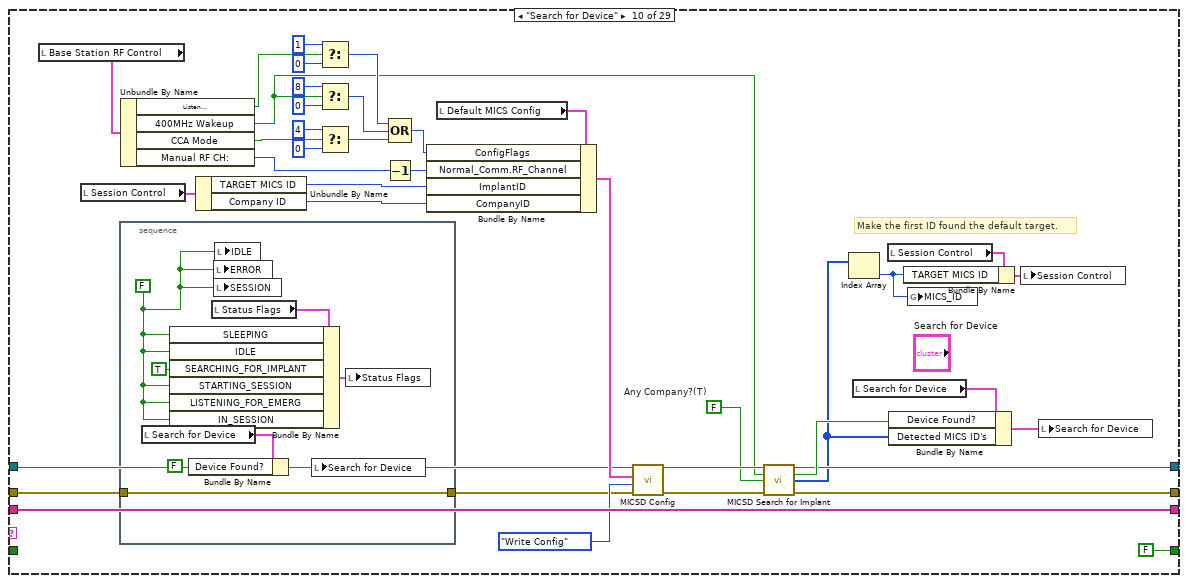
[diagram p12: hidden frame]
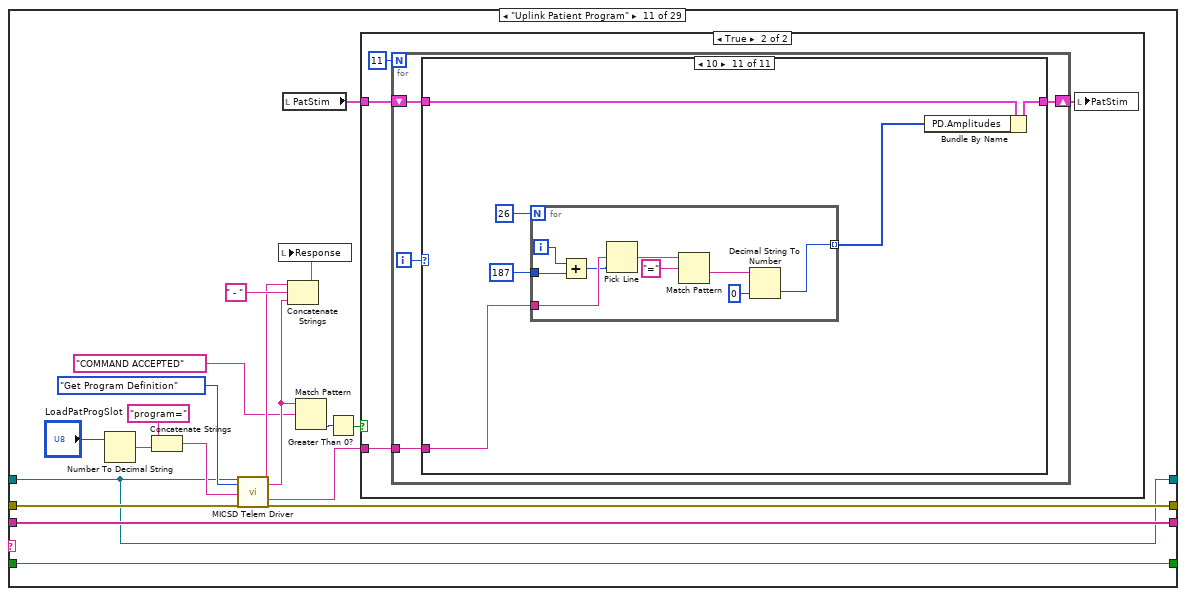
[diagram p13: hidden frame]
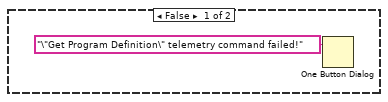
[diagram p14: hidden frame]
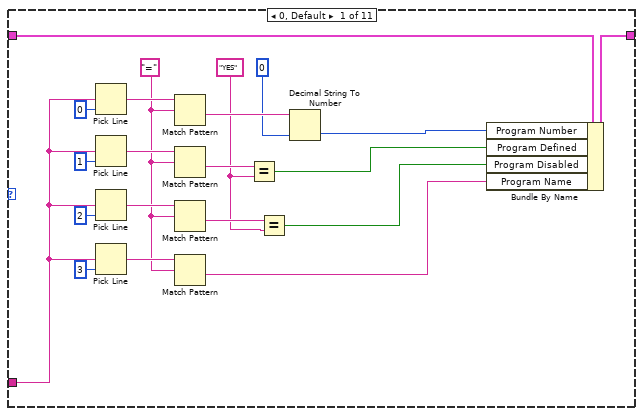
[diagram p15: hidden frame]
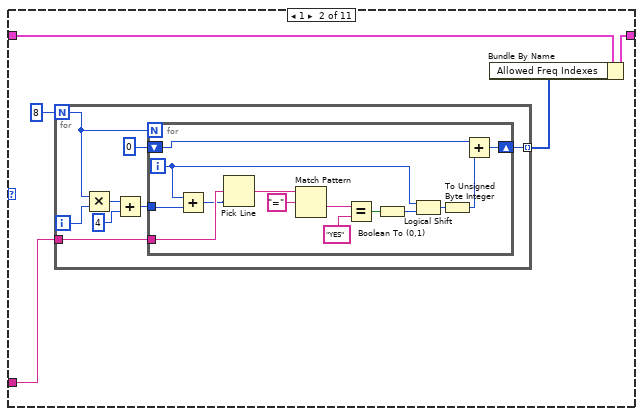
[diagram p16: hidden frame]
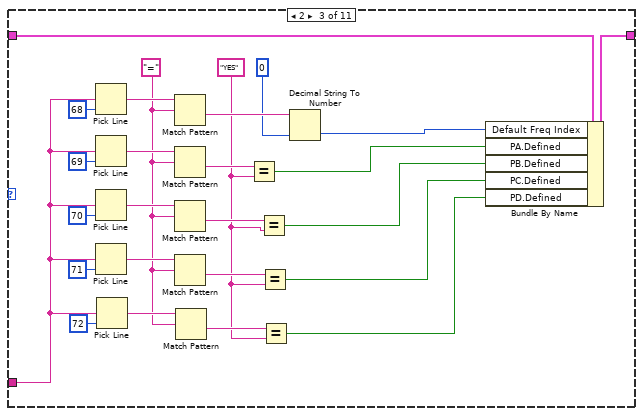
[diagram p17: hidden frame]
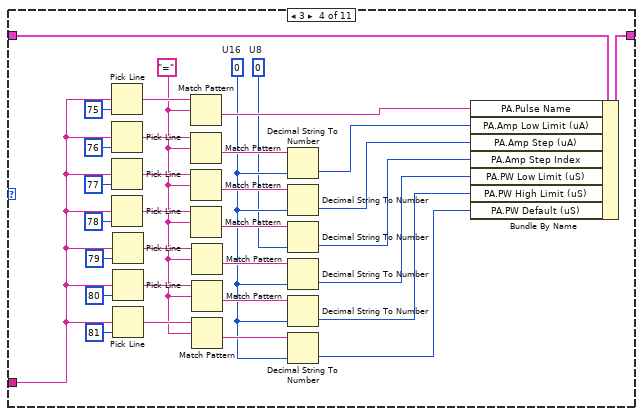
[diagram p18: hidden frame]
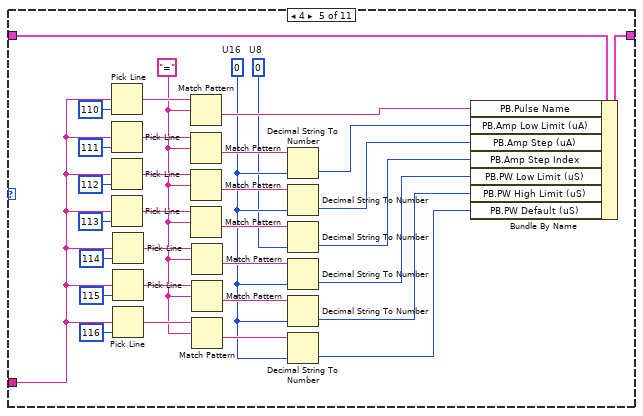
[diagram p19: hidden frame]
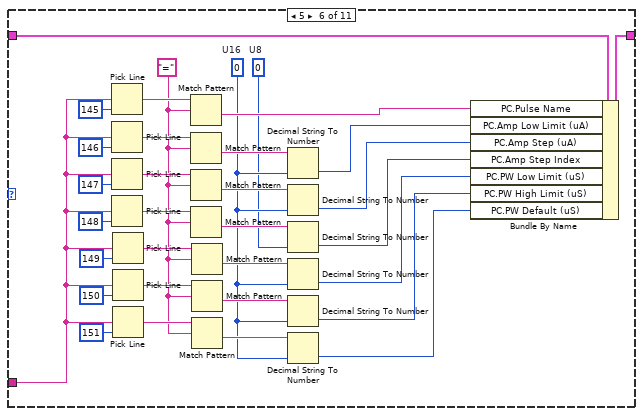
[diagram p20: hidden frame]
diagram:
  n1 = call-poly "VISA Configure Serial Port"("VISA resource name"="VISA Resource Name", "Enable Termination\nChar (T)"=FALSE ("Enable Termination\nChar (T)"), "baud rate (9600)"=u32 230400, "error in (no error)"="error in (no error)") -> ("VISA resource name out"=w4:refnum<visa-resource-name>, "error out"=w5:errorcluster)  [unwired: 10 in]
  n2 = while {
    shift-right: [w25] -> w12
    shift-left: w5 -> [w18]
    shift-right: [w16] -> _
    shift-left: FALSE -> [w26]
    tunnel: w4 -> [w24]
    shift-right: [w19] -> _
    shift-left: string[] ["Initialize", "Get Status"] -> [w21]
    tunnel: "Top of Loop" -> [w22]
    tunnel: [w14] -> w1
    stop <- w17 stop-if-true
    n3 = call "State Select.vi"("State In"=w22, "error in (no error)"=w18, "States Array In"=w21) -> ("State Out"=w23:string, "States Array Out"=w20:string[])  [unwired: 7 in]
    n4 = case shown="\"Initialize\"" w23 {
      tunnel: w26 -> [w35 w66 _ w107 w155 w187 w216 w230 w244 _ w310 w603 w842 w869 w1009 w1023 w1034 w1045 w1053 w1063 w1079 w1098 w1117 w1130 w1143 w1157 w1176 w1182 w1197]
      tunnel: [w35 w66 FALSE w107 w155 w187 w216 w230 w244 FALSE w310 w603 w842 w869 w1009 w1023 w1034 w1045 w1053 w1063 w1079 w1098 w1117 w1130 w1143 w1157 w1176 w1182 w1197] -> w16
      tunnel: w18 -> [w33 w62 w74 w99 w138 w185 w214 w228 w242 w278 w307 w605 w832 w867 w1007 w1021 w1032 w1043 w1051 w1055 w1075 w1096 w1115 w1129 w1142 w1156 w1174 w1179 w1194]
      tunnel: [w30 w65 w73 w105 w138 w183 w212 w226 w240 w281 w308 w605 w822 w867 w1006 w1020 w1031 w1042 w1049 w1055 w1075 w1094 w1111 w1124 w1140 w1150 w1172 w1177 w1192] -> w25
      tunnel: w24 -> [w28 w60 w72 w98 w139 w163 w192 w224 w238 w251 w299 w594 w835 w866 w999 w1014 w1025 w1036 w1050 w1061 w1077 w1095 w1114 w1128 w1141 w1155 w1173 w1180 w1193]
      tunnel: w20 -> [w36 w67 w75 w108 w156 w186 w215 w229 w243 w282 w309 w600 w834 w868 w1008 w1022 w1033 w1044 w1052 w1062 w1078 w1097 w1116 w1131 w1144 w1158 w1175 w1181 w1196]
      tunnel: [w36 w67 w75 w108 w156 w186 w215 w229 w243 w282 w309 w593 w834 w868 w1008 w1022 w1033 w1044 w1052 w1062 w1078 w1097 w1116 w1131 w1144 w1158 w1175 w1181 w1196] -> w19
      tunnel: [w28 w60 w71 w81 w144 w163 w192 w224 w238 w277 w299 w594 w821 w866 w999 w1014 w1025 w1036 w1048 w1061 w1077 w1093 w1113 w1123 w1139 w1154 w1171 w1178 w1183] -> w14
      frame "Error", Default {
        n5 = stacked-sequence {
          tunnel: w33 -> [w43]
          tunnel: [w43] -> w32
          frame #0 {
            w42 = TRUE ("Visible")
            n6 = property on="Error Flag" class="Str"("Visible"=w42) -> ()  [unwired: 2 in, 2 out]
            n7 = property on="Clear Error" class="Bool"("Visible"=w42) -> ()  [unwired: 2 in, 2 out]
            n8 = Wait (ms)(milliseconds to wait=u32 500) -> ()  [unwired: 1 out]
          }
        }
        n9 = local write "Tab Control"(T1."Session" ("Tab Control")) -> ()
        n10 = Select(t=errorcluster {"status"=FALSE, "code"=0, "source"=""}, s="Clear Error", f=w32) -> (s? t:f=w31:errorcluster)
        n11 = stacked-sequence {
          tunnel: w31 -> [w40]
          tunnel: [w40] -> w30
          tunnel: "Clear Error" -> [w38]
          frame #0 {
            n12 = Not(x=w38) -> (.not. x?=w37:bool)
            n13 = Wait (ms)(milliseconds to wait=u32 500) -> ()  [unwired: 1 out]
            n14 = property on="Clear Error" class="Bool"("Visible"=w37) -> ()  [unwired: 2 in, 2 out]
            n15 = property on="Error Flag" class="Str"("Visible"=FALSE) -> ()  [unwired: 2 in, 2 out]
          }
        }
      }
      frame "Telem Driver" {
        n16 = flat-sequence {
          tunnel: w62 -> [w68]
          tunnel: [w68] -> w61
          frame #0 {
            w69 = ""
            w70 = FALSE
            n17 = local write "bChecksum Valid"(w70) -> ()
            n18 = local write "tChecksum Valid"(w70) -> ()
            n19 = local write "Response Token"(w69) -> ()
            n20 = local write "Response Code"(w69) -> ()
            n21 = local write "Response"(w69) -> ()
            n22 = local write "Data"(w69) -> ()
          }
        }
        n23 = Unbundle By Name("Session Control") -> ("TARGET MICS ID"=w45:u32)
        n24 = Bundle By Name(cluster=T12 {"Command"=enum."Get xPG Status", "Function"=enum."Downlink Only", "MICS_ID"=0, "EXID"=16773121, "Use Local"=FALSE, "Transceive Delay mS"=200.0, "CP_DATA IN"=[], "Parameters"=""} ("Input"), "Command"="Command", "Function"=T13."Transceive (DN -> UP)", "Parameters"="Parameters", "CP_DATA IN"="CP_DATA IN", "MICS_ID"=w45) -> (w54:T12)
        n25 = call "Zarlink Telemetry.vi"("error in (no error)"=w61, "Input"=w54, "MICS Dongle Address"=w60) -> ("error out"=w65:errorcluster, "Output"=w53:T16)  [unwired: 6 in, 1 out]
        n26 = Unbundle By Name(w53) -> ("Response Token"=w48:string, "Response Code"=w47:string, "bChecksum Valid"=→"bChecksum Valid":bool, "tChecksum Valid"=→"tChecksum Valid":bool, "Data"=→"Data":string, "CP_DATA OUT"=→"CP_DATA OUT":u8[])
        "Response Token" <- w48
        "Response Code" <- w47
        n27 = Concatenate Strings(w48, " - ", w47) -> (w64:string)
        n28 = local write "Response"(w64) -> ()
      }
      frame "Close Session" {
        n29 = call "MICSD Abort.vi"("error in (no error)"=w74, "VISA Resource Name"=w72) -> ("error out"=w73:errorcluster, "dup VISA Resource Name"=w71:refnum<visa-resource-name>)  [unwired: 8 in]
      }
      frame "Open Session" {
        n30 = local read "Base Station RF Control"() -> (w89:T2)
        n31 = local read "Session Control"() -> (w80:T4)
        n32 = Unbundle By Name(w80) -> ("Calibrate Antenna on \"Open Session\"?"=w79:bool)
        n33 = Unbundle By Name(w89) -> ("Listen\nfor\nEmergency"=w83:bool, "400MHz Wakeup"=w82:bool, "CCA Mode"=w88:bool, "Manual RF CH:"=w87:u8)
        n34 = Unbundle By Name(w80) -> ("TARGET MICS ID"=w100:u32, "Company ID"=w101:u8)
        n35 = Decrement(x=w87) -> (x-1=w97:u8)
        n36 = Select(t=u8 1, s=w83, f=u8 0) -> (s? t:f=w84:u8)
        n37 = Select(t=u8 8, s=w82, f=u8 0) -> (s? t:f=w91:u8)
        n38 = Select(t=u8 4, s=w88, f=u8 0) -> (s? t:f=w90:u8)
        n39 = case shown="True" w79 {
          tunnel: [w109 w111] -> w77
          tunnel: w99 -> [w109 w118]
          tunnel: w98 -> [w110 w117]
          tunnel: w97 -> [_ w116]
          tunnel: [w110 w113] -> w78
          frame False {
            # "DO NOT\nCALIBRATE ANTENNA!"
          }
          frame True {
            # "CALIBRATE ANTENNA\nFOR INTENDED CHANNEL"
            n40 = call "MICSD Calibrate.vi"("VISA Resource Name"=w117, "CalSelect1"=u8 64, "Channel"=w116, "error in (no error)"=w118) -> ("dup VISA Resource Name"=w114:refnum<visa-resource-name>, "error out"=w112:errorcluster)  [unwired: 10 in]
            n41 = stacked-sequence {
              tunnel: w114 -> [w120]
              tunnel: [w120] -> w113
              tunnel: w112 -> [w119]
              tunnel: [w119] -> w111
              frame #0 {
                n42 = Wait (ms)(milliseconds to wait=u32 200) -> ()  [unwired: 1 out]
              }
            }
          }
        }
        n43 = Compound Arithmetic op=OR(w84, w91, w90) -> (w92:u8)
        n44 = Bundle By Name(cluster="Default MICS Config", "ConfigFlags"=w92, "Normal_Comm.RF_Channel"=w97, "ImplantID"=w100, "CompanyID"=w101) -> (w102:T11)
        n45 = call "MICSD Config.vi"("error in (no error)"=w77, "Function"=enum16{"Write Config", "Read Config"}."Write Config", "MICS_Config_In"=w102, "VISA Resource Name"=w78) -> ("error out"=w106:errorcluster, "dup VISA Resource Name"=w81:refnum<visa-resource-name>)  [unwired: 5 in, 1 out]
        n46 = case shown="False" w83 {
          tunnel: w106 -> [w126 w137]
          tunnel: w81 -> [w125 _]
          tunnel: [w122 w137] -> w105
          frame False {
            # "Listen for Emergency was not selected"
            n47 = call "MICSD Start Session.vi"("error in (no error)"=w126, "VISA Resource Name"=w125) -> ("error out"=w124:errorcluster, "dup VISA Resource Name"=w123:refnum<visa-resource-name>)  [unwired: 8 in]
            n48 = while {
              tunnel: w123 -> [w135]
              shift-right: [w134] -> w122
              shift-left: w124 -> [w136]
              i -> [w129]
              stop <- w130 stop-if-true
              n49 = Wait (ms)(milliseconds to wait=u32 100) -> ()  [unwired: 1 out]
              n50 = call "MICSD Status.vi"("VISA Resource Name"=w135, "error in (no error)"=w136) -> ("Status Flags"=w127:T8, "error out"=w134:errorcluster)  [unwired: 7 in, 5 out]
              n51 = Unbundle By Name(w127) -> ("IN_SESSION"=w132:bool)
              n52 = Greater?(x=w129, y=60) -> (0:w131:bool)
              n53 = local write "Status Flags"(w127) -> ()
              n54 = Or(x=w132, y=w131) -> (x .or. y?=w130:bool)
            }
          }
          frame True {
            # "Listen for Emergency was selected, do not open a session"
          }
        }
      }
      frame "Initialize" {
        w151 = FALSE ("Visible")
        w153 = FALSE
        w154 = T3 {"Search for Device"=FALSE, "Device Found?"=FALSE, "Detected MICS ID's"=[]}  # Search for Device
        w141 = T17 {"Open Session"=FALSE, "Close Session"=FALSE, "TARGET MICS ID"=0, "EXID"=16773121, "Company ID"=187, TRUE}  # Session Control
        n55 = global read "MICS_ID Global.vi" "MICS_ID"() -> (w140:u32)
        n56 = Bundle By Name(cluster=w141, "TARGET MICS ID"=w140) -> (w142:T17)
        n57 = local write "Base Station RF Control"(T2 {"CCA Mode"=FALSE, "Manual RF CH:"=2, "Base Station CCA Results"=[], "Update CCA"=FALSE, "RSSI Measurement"=0, "Use Averaging?"=TRUE, "400MHz Wakeup"=FALSE, "Listen\nfor\nEmergency"=FALSE} ("Base Station RF Control")) -> ()
        n58 = local write "Search for Device"(w154) -> ()
        n59 = local write "Session Control"(w142) -> ()
        n60 = flat-sequence {
          tunnel: w139 -> [w158]
          tunnel: [w158] -> w144
          frame #0 {
            n61 = Wait (ms)(milliseconds to wait=u32 100) -> ()  [unwired: 1 out]
          }
        }
        n62 = local write "Default MICS Config"(T11 {"ConfigFlags"=0, "ImplantID"=1048576, "CompanyID"=187, "Normal_Comm"={"RF_Channel"=4, "UserData"=0, "TX_Mod"=0, "RX_Mod"=0, "RX_BlockSize"=15, "BlockPerPack"=31, "TX_BlockSize"=15}, "Emerg_Comm"={"RF_Channel"=4, "UserData"=0, "TX_Mod"=0, "RX_Mod"=0, "TX_BlockSize"=15, "BlockPerPack"=31, "RX_BlockSize"=15}, "ImplantRev"=4, "245TX_PowerCal"=0, "245TX_Power"=10, "CCA_RSSI_Thresholds"={"ch0"=2650, "ch1"=2650, "ch2"=2650, "ch3"=2650, "ch4"=2650, "ch5"=2650, "ch6"=2650, "ch7"=2650, "ch8"=2650, "ch9"=2650}} ("MICS_Config_In")) -> ()
        n63 = local write "ERROR"(w153) -> ()
        n64 = local write "SESSION"(w153) -> ()
        n65 = local write "IDLE"(w153) -> ()
        n66 = local write "Tab Control"(T1."Session" ("Tab Control")) -> ()
        n67 = property on="Error Flag" class="Str"("Visible"=w151) -> ()  [unwired: 2 in, 2 out]
        n68 = property on="Clear Error" class="Bool"("Visible"=w151) -> ()  [unwired: 2 in, 2 out]
        n69 = local read "PatStim"() -> (w147:T10)
        n70 = Bundle By Name(cluster=w147, "label.freqindex"=string[] ["1-7", "8-15", "16-23", "24-31", "32-39", "40-47", "48-55", "56-63"]) -> (w148:T10)
        n71 = local write "PatStim"(w148) -> ()
        "Error Flag" <- "ERROR" ("Error Flag")
        "Busy Flag" <- "Busy..." ("Busy Flag")
      }
      frame "Increment Program Ampl" {
        n72 = call "MICSD Telem Driver.vi"("VISA Resource Name"=w163, "Command"=Typedef_Command_List."Increment Program Amplitude", "error in (no error)"=w185) -> ("Response Token"=w160:string, "Response Code"=w159:string, "Data"=w164:string, "error out"=w183:errorcluster)  [unwired: 10 in, 3 out]
        n73 = Concatenate Strings(w160, " - ", w159) -> (w161:string)
        n74 = Pick Line(multi-line string=w164, line index=4) -> (output string=w180:string)  [unwired: 1 in]
        n75 = local write "Response"(w161) -> ()
        n76 = Match Pattern(string=w180, regular expression="=") -> (after substring=w178:string)  [unwired: 1 in, 3 out]
        n77 = Match Pattern(string=w178, regular expression=",") -> (before substring=w177:string, after substring=w176:string)  [unwired: 1 in, 2 out]
        n78 = Match Pattern(string=w176, regular expression=",") -> (before substring=w172:string, after substring=w173:string)  [unwired: 1 in, 2 out]
        n79 = Match Pattern(string=w173, regular expression=",") -> (before substring=w171:string, after substring=w170:string)  [unwired: 1 in, 2 out]
        n80 = Decimal String To Number(string=w177) -> (number=w169:i32)  [unwired: 2 in, 1 out]
        n81 = Decimal String To Number(string=w172) -> (number=w168:i32)  [unwired: 2 in, 1 out]
        n82 = Decimal String To Number(string=w171) -> (number=w167:i32)  [unwired: 2 in, 1 out]
        n83 = Decimal String To Number(string=w170) -> (number=w166:i32)  [unwired: 2 in, 1 out]
        n84 = Build Array(w169, w168, w167, w166) -> (w165:i32[])
        n85 = local write "ProgAmpls"(w165) -> ()
      }
      frame "Decrement Program Ampl" {
        n86 = call "MICSD Telem Driver.vi"("VISA Resource Name"=w192, "Command"=Typedef_Command_List."Decrement Program Amplitude", "error in (no error)"=w214) -> ("Response Token"=w189:string, "Response Code"=w190:string, "Data"=w193:string, "error out"=w212:errorcluster)  [unwired: 10 in, 3 out]
        n87 = Concatenate Strings(w189, " - ", w190) -> (w188:string)
        n88 = Pick Line(multi-line string=w193, line index=4) -> (output string=w209:string)  [unwired: 1 in]
        n89 = local write "Response"(w188) -> ()
        n90 = Match Pattern(string=w209, regular expression="=") -> (after substring=w207:string)  [unwired: 1 in, 3 out]
        n91 = Match Pattern(string=w207, regular expression=",") -> (before substring=w206:string, after substring=w205:string)  [unwired: 1 in, 2 out]
        n92 = Match Pattern(string=w205, regular expression=",") -> (before substring=w201:string, after substring=w202:string)  [unwired: 1 in, 2 out]
        n93 = Match Pattern(string=w202, regular expression=",") -> (before substring=w200:string, after substring=w199:string)  [unwired: 1 in, 2 out]
        n94 = Decimal String To Number(string=w206) -> (number=w198:i32)  [unwired: 2 in, 1 out]
        n95 = Decimal String To Number(string=w201) -> (number=w197:i32)  [unwired: 2 in, 1 out]
        n96 = Decimal String To Number(string=w200) -> (number=w196:i32)  [unwired: 2 in, 1 out]
        n97 = Decimal String To Number(string=w199) -> (number=w195:i32)  [unwired: 2 in, 1 out]
        n98 = Build Array(w198, w197, w196, w195) -> (w194:i32[])
        n99 = local write "ProgAmpls"(w194) -> ()
      }
      frame "Increment Program Freq" {
        n100 = call "MICSD Telem Driver.vi"("VISA Resource Name"=w224, "Command"=Typedef_Command_List."Increment Program Frequency", "error in (no error)"=w228) -> ("Response Token"=w221:string, "Response Code"=w222:string, "Data"=w217:string, "error out"=w226:errorcluster)  [unwired: 10 in, 3 out]
        n101 = Concatenate Strings(w221, " - ", w222) -> (w220:string)
        n102 = local write "Response"(w220) -> ()
        n103 = Match Pattern(string=w217, regular expression="=") -> (after substring=w219:string)  [unwired: 1 in, 3 out]
        n104 = Decimal String To Number(string=w219) -> (number=w218:i32)  [unwired: 2 in, 1 out]
        n105 = local write "Freq Index"(w218) -> ()
      }
      frame "Decrement Program Freq" {
        n106 = call "MICSD Telem Driver.vi"("VISA Resource Name"=w238, "Command"=Typedef_Command_List."Decrement Program Frequency", "error in (no error)"=w242) -> ("Response Token"=w235:string, "Response Code"=w236:string, "Data"=w231:string, "error out"=w240:errorcluster)  [unwired: 10 in, 3 out]
        n107 = Concatenate Strings(w235, " - ", w236) -> (w234:string)
        n108 = local write "Response"(w234) -> ()
        n109 = Match Pattern(string=w231, regular expression="=") -> (after substring=w233:string)  [unwired: 1 in, 3 out]
        n110 = Decimal String To Number(string=w233) -> (number=w232:i32)  [unwired: 2 in, 1 out]
        n111 = local write "Freq Index"(w232) -> ()
      }
      frame "Search for Device" {
        w247 = FALSE  # Any Company?(T)
        # "Make the first ID found the default target."
        n112 = local read "Base Station RF Control"() -> (w259:T2)
        n113 = local read "Session Control"() -> (w270:T4)
        n114 = stacked-sequence {
          tunnel: w278 -> [w289]
          tunnel: [w289] -> w250
          frame #0 {
            w284 = FALSE ("Device Found?")
            n115 = local read "Search for Device"() -> (w290:T3)
            n116 = Bundle By Name(cluster=w290, "Device Found?"=FALSE) -> (w291:T3)
            n117 = local read "Status Flags"() -> (w287:T8)
            n118 = Bundle By Name(cluster=w287, "SLEEPING"=w284, "IDLE"=w284, "SEARCHING_FOR_IMPLANT"=TRUE ("Device Found?"), "STARTING_SESSION"=w284, "LISTENING_FOR_EMERG"=w284, "IN_SESSION"=w284) -> (w286:T8)
            n119 = local write "ERROR"(w284) -> ()
            n120 = local write "SESSION"(w284) -> ()
            n121 = local write "IDLE"(w284) -> ()
            n122 = local write "Search for Device"(w291) -> ()
            n123 = local write "Status Flags"(w286) -> ()
          }
        }
        n124 = Unbundle By Name(w259) -> ("Listen\nfor\nEmergency"=w253:bool, "400MHz Wakeup"=w246:bool, "CCA Mode"=w258:bool, "Manual RF CH:"=w257:u8)
        n125 = Unbundle By Name(w270) -> ("TARGET MICS ID"=w268:u32, "Company ID"=w269:u8)
        n126 = Select(t=u8 1, s=w253, f=u8 0) -> (s? t:f=w254:u8)
        n127 = Select(t=u8 8, s=w246, f=u8 0) -> (s? t:f=w261:u8)
        n128 = Select(t=u8 4, s=w258, f=u8 0) -> (s? t:f=w260:u8)
        n129 = Decrement(x=w257) -> (x-1=w267:u8)
        n130 = Compound Arithmetic op=OR(w254, w261, w260) -> (w262:u8)
        n131 = local read "Default MICS Config"() -> (w252:T11)
        n132 = Bundle By Name(cluster=w252, "ConfigFlags"=w262, "Normal_Comm.RF_Channel"=w267, "ImplantID"=w268, "CompanyID"=w269) -> (w271:T11)
        n133 = call "MICSD Config.vi"("error in (no error)"=w250, "Function"=enum16{"Write Config", "Read Config"}."Write Config", "MICS_Config_In"=w271, "VISA Resource Name"=w251) -> ("error out"=w248:errorcluster, "dup VISA Resource Name"=w249:refnum<visa-resource-name>)  [unwired: 5 in, 1 out]
        n134 = call "MICSD Search for Implant.vi"("VISA Resource Name"=w249, "Enable Watchdog?(T)"=w246, "Any Company?(T)"=w247, "error in (no error)"=w248) -> ("dup VISA Resource Name"=w277:refnum<visa-resource-name>, "Device Found?"=w280:bool, "Detected MICS IDs"=w275:u32[], "error out"=w281:errorcluster)  [unwired: 8 in]
        n135 = Index Array(array=w275) -> (element=w245:u32)  [unwired: 1 in]
        n136 = local read "Search for Device"() -> (w279:T3)
        n137 = local read "Session Control"() -> (w274:T4)
        n138 = Bundle By Name(cluster=w279, "Device Found?"=w280, "Detected MICS ID's"=w275) -> (w276:T3)
        n139 = Bundle By Name(cluster=w274, "TARGET MICS ID"=w245) -> (w273:T4)
        n140 = global write "MICS_ID Global.vi" "MICS_ID"(w245) -> ()
        n141 = local write "Session Control"(w273) -> ()
        n142 = local write "Search for Device"(w276) -> ()
      }
      frame "Uplink Patient Program" {
        n143 = Number To Decimal String(number="LoadPatProgSlot") -> (decimal integer string=w304:string)  [unwired: 1 in]
        n144 = Concatenate Strings("program=", w304) -> (w302:string)
        n145 = call "MICSD Telem Driver.vi"("VISA Resource Name"=w299, "Command"=Typedef_Command_List."Get Program Definition", "Parameters"=w302, "error in (no error)"=w307) -> ("Response Token"=w296:string, "Response Code"=w295:string, "Data"=w301:string, "error out"=w308:errorcluster)  [unwired: 9 in, 3 out]
        n146 = local read "PatStim"() -> (w300:T10)
        n147 = Concatenate Strings(w296, " - ", w295) -> (w297:string)
        n148 = local write "Response"(w297) -> ()
        n149 = Match Pattern(string=w295, regular expression="COMMAND ACCEPTED" ("Response Code")) -> (offset past match=w293:i32)  [unwired: 1 in, 3 out]
        n150 = Greater Than 0?(x=w293) -> (x > 0?=w292:bool)
        n151 = case shown="True" w292 {
          tunnel: w301 -> [_ w313]
          tunnel: w300 -> [_ w314]
          frame False {
            n152 = One Button Dialog(message="\"Get Program Definition\" telemetry command failed!") -> ()  [unwired: 1 in, 1 out]
          }
          frame True {
            n153 = for {
              N: 11 -> [_]
              shift-right: [w316] -> w315
              shift-left: w314 -> [w318]
              tunnel: w313 -> [w317]
              i -> [w319]
              n154 = case shown="10" w319 {
                tunnel: w318 -> [w325 w343 w381 w418 w451 w484 w517 w531 w546 w561 w576]
                tunnel: w317 -> [w331 w344 w369 w410 w443 w476 w509 w529 w544 w559 w574]
                tunnel: [w324 w342 w380 w417 w450 w483 w516 w530 w545 w560 w575] -> w316
                frame 0, Default {
                  w326 = "YES"
                  w332 = "="
                  n155 = Pick Line(multi-line string=w331, line index=0) -> (output string=w339:string)  [unwired: 1 in]
                  n156 = Pick Line(multi-line string=w331, line index=1) -> (output string=w337:string)  [unwired: 1 in]
                  n157 = Pick Line(multi-line string=w331, line index=2) -> (output string=w335:string)  [unwired: 1 in]
                  n158 = Pick Line(multi-line string=w331, line index=3) -> (output string=w333:string)  [unwired: 1 in]
                  n159 = Match Pattern(string=w339, regular expression=w332) -> (after substring=w330:string)  [unwired: 1 in, 3 out]
                  n160 = Match Pattern(string=w337, regular expression=w332) -> (after substring=w328:string)  [unwired: 1 in, 3 out]
                  n161 = Match Pattern(string=w335, regular expression=w332) -> (after substring=w327:string)  [unwired: 1 in, 3 out]
                  n162 = Match Pattern(string=w333, regular expression=w332) -> (after substring=w323:string)  [unwired: 1 in, 3 out]
                  n163 = Equal?(x=w328, y=w326) -> (x = y?=w321:bool)
                  n164 = Equal?(x=w327, y=w326) -> (x = y?=w322:bool)
                  n165 = Decimal String To Number(string=w330, default (0L)=u8 0 ("line index")) -> (number=w320:u8)  [unwired: 1 in, 1 out]
                  n166 = Bundle By Name(cluster=w325, "Program Number"=w320, "Program Defined"=w321, "Program Disabled"=w322, "Program Name"=w323) -> (w324:T10)
                }
                frame 1 {
                  n167 = for {
                    N: 8 -> [w349]
                    tunnel: w344 -> [w352]
                    tunnel: [w350] -> w341 mode=indexing
                    i -> [w353]
                    n168 = Multiply(x=w349, y=w353) -> (x*y=w348:i32)
                    n169 = Add(x=w348, y=4) -> (x+y=w346:i32)
                    n170 = for {
                      N: w349 -> [_]
                      tunnel: w346 -> [w355]
                      tunnel: w352 -> [w364]
                      shift-right: [w359] -> w350
                      shift-left: u8 0 ("y") -> [w360]
                      i -> [w354]
                      n171 = Add(x=w354, y=w355) -> (x+y=w356:i32)
                      n172 = Pick Line(multi-line string=w364, line index=w356) -> (output string=w367:string)  [unwired: 1 in]
                      n173 = Match Pattern(string=w367, regular expression="=") -> (after substring=w366:string)  [unwired: 1 in, 3 out]
                      n174 = Equal?(x=w366, y="YES") -> (x = y?=w362:bool)
                      n175 = Boolean To (0,1)(Boolean=w362) -> (0, 1=w361:i16)
                      n176 = Logical Shift(y=w354, x=w361) -> (x << y=w358:i16)
                      n177 = To Unsigned Byte Integer(number=w358) -> (unsigned 8bit integer=w357:u8)
                      n178 = Add(x=w360, y=w357) -> (x+y=w359:u8)
                    }
                  }
                  n179 = Bundle By Name(cluster=w343, "Allowed Freq Indexes"=w341) -> (w342:T10)
                }
                frame 2 {
                  w370 = "YES"
                  w371 = "="
                  n180 = Pick Line(multi-line string=w369, line index=68) -> (output string=w392:string)  [unwired: 1 in]
                  n181 = Pick Line(multi-line string=w369, line index=69) -> (output string=w390:string)  [unwired: 1 in]
                  n182 = Pick Line(multi-line string=w369, line index=70) -> (output string=w388:string)  [unwired: 1 in]
                  n183 = Pick Line(multi-line string=w369, line index=71) -> (output string=w386:string)  [unwired: 1 in]
                  n184 = Pick Line(multi-line string=w369, line index=72) -> (output string=w373:string)  [unwired: 1 in]
                  n185 = Match Pattern(string=w392, regular expression=w371) -> (after substring=w385:string)  [unwired: 1 in, 3 out]
                  n186 = Match Pattern(string=w390, regular expression=w371) -> (after substring=w383:string)  [unwired: 1 in, 3 out]
                  n187 = Match Pattern(string=w388, regular expression=w371) -> (after substring=w382:string)  [unwired: 1 in, 3 out]
                  n188 = Match Pattern(string=w386, regular expression=w371) -> (after substring=w376:string)  [unwired: 1 in, 3 out]
                  n189 = Match Pattern(string=w373, regular expression=w371) -> (after substring=w372:string)  [unwired: 1 in, 3 out]
                  n190 = Equal?(x=w383, y=w370) -> (x = y?=w378:bool)
                  n191 = Equal?(x=w382, y=w370) -> (x = y?=w379:bool)
                  n192 = Equal?(x=w376, y=w370) -> (x = y?=w375:bool)
                  n193 = Equal?(x=w372, y=w370) -> (x = y?=w368:bool)
                  n194 = Decimal String To Number(string=w385, default (0L)=u8 0 ("line index")) -> (number=w377:u8)  [unwired: 1 in, 1 out]
                  n195 = Bundle By Name(cluster=w381, "Default Freq Index"=w377, "PA.Defined"=w378, "PB.Defined"=w379, "PC.Defined"=w375, "PD.Defined"=w368) -> (w380:T10)
                }
                frame 3 {
                  w401 = u16 0  # U16
                  w400 = u8 0  # U8
                  w409 = "="
                  n196 = Pick Line(multi-line string=w410, line index=75) -> (output string=w425:string)  [unwired: 1 in]
                  n197 = Pick Line(multi-line string=w410, line index=76) -> (output string=w423:string)  [unwired: 1 in]
                  n198 = Pick Line(multi-line string=w410, line index=77) -> (output string=w421:string)  [unwired: 1 in]
                  n199 = Pick Line(multi-line string=w410, line index=78) -> (output string=w419:string)  [unwired: 1 in]
                  n200 = Pick Line(multi-line string=w410, line index=79) -> (output string=w415:string)  [unwired: 1 in]
                  n201 = Pick Line(multi-line string=w410, line index=80) -> (output string=w413:string)  [unwired: 1 in]
                  n202 = Pick Line(multi-line string=w410, line index=81) -> (output string=w411:string)  [unwired: 1 in]
                  n203 = Match Pattern(string=w425, regular expression=w409) -> (after substring=w402:string)  [unwired: 1 in, 3 out]
                  n204 = Match Pattern(string=w423, regular expression=w409) -> (after substring=w408:string)  [unwired: 1 in, 3 out]
                  n205 = Match Pattern(string=w421, regular expression=w409) -> (after substring=w403:string)  [unwired: 1 in, 3 out]
                  n206 = Match Pattern(string=w419, regular expression=w409) -> (after substring=w404:string)  [unwired: 1 in, 3 out]
                  n207 = Match Pattern(string=w415, regular expression=w409) -> (after substring=w405:string)  [unwired: 1 in, 3 out]
                  n208 = Match Pattern(string=w413, regular expression=w409) -> (after substring=w406:string)  [unwired: 1 in, 3 out]
                  n209 = Match Pattern(string=w411, regular expression=w409) -> (after substring=w407:string)  [unwired: 1 in, 3 out]
                  n210 = Decimal String To Number(string=w408, default (0L)=w401) -> (number=w399:u16)  [unwired: 1 in, 1 out]
                  n211 = Decimal String To Number(string=w403, default (0L)=w401) -> (number=w398:u16)  [unwired: 1 in, 1 out]
                  n212 = Decimal String To Number(string=w404, default (0L)=w400) -> (number=w397:u8)  [unwired: 1 in, 1 out]
                  n213 = Decimal String To Number(string=w405, default (0L)=w401) -> (number=w396:u16)  [unwired: 1 in, 1 out]
                  n214 = Decimal String To Number(string=w406, default (0L)=w401) -> (number=w395:u16)  [unwired: 1 in, 1 out]
                  n215 = Decimal String To Number(string=w407, default (0L)=w401) -> (number=w394:u16)  [unwired: 1 in, 1 out]
                  n216 = Bundle By Name(cluster=w418, "PA.Pulse Name"=w402, "PA.Amp Low Limit (uA)"=w399, "PA.Amp Step (uA)"=w398, "PA.Amp Step Index"=w397, "PA.PW Low Limit (uS)"=w396, "PA.PW High Limit (uS)"=w395, "PA.PW Default (uS)"=w394) -> (w417:T10)
                }
                frame 4 {
                  w434 = u16 0  # U16
                  w433 = u8 0  # U8
                  w442 = "="
                  n217 = Pick Line(multi-line string=w443, line index=110) -> (output string=w458:string)  [unwired: 1 in]
                  n218 = Pick Line(multi-line string=w443, line index=111) -> (output string=w456:string)  [unwired: 1 in]
                  n219 = Pick Line(multi-line string=w443, line index=112) -> (output string=w454:string)  [unwired: 1 in]
                  n220 = Pick Line(multi-line string=w443, line index=113) -> (output string=w452:string)  [unwired: 1 in]
                  n221 = Pick Line(multi-line string=w443, line index=114) -> (output string=w448:string)  [unwired: 1 in]
                  n222 = Pick Line(multi-line string=w443, line index=115) -> (output string=w446:string)  [unwired: 1 in]
                  n223 = Pick Line(multi-line string=w443, line index=116) -> (output string=w444:string)  [unwired: 1 in]
                  n224 = Match Pattern(string=w458, regular expression=w442) -> (after substring=w435:string)  [unwired: 1 in, 3 out]
                  n225 = Match Pattern(string=w456, regular expression=w442) -> (after substring=w441:string)  [unwired: 1 in, 3 out]
                  n226 = Match Pattern(string=w454, regular expression=w442) -> (after substring=w436:string)  [unwired: 1 in, 3 out]
                  n227 = Match Pattern(string=w452, regular expression=w442) -> (after substring=w437:string)  [unwired: 1 in, 3 out]
                  n228 = Match Pattern(string=w448, regular expression=w442) -> (after substring=w438:string)  [unwired: 1 in, 3 out]
                  n229 = Match Pattern(string=w446, regular expression=w442) -> (after substring=w439:string)  [unwired: 1 in, 3 out]
                  n230 = Match Pattern(string=w444, regular expression=w442) -> (after substring=w440:string)  [unwired: 1 in, 3 out]
                  n231 = Decimal String To Number(string=w441, default (0L)=w434) -> (number=w432:u16)  [unwired: 1 in, 1 out]
                  n232 = Decimal String To Number(string=w436, default (0L)=w434) -> (number=w431:u16)  [unwired: 1 in, 1 out]
                  n233 = Decimal String To Number(string=w437, default (0L)=w433) -> (number=w430:u8)  [unwired: 1 in, 1 out]
                  n234 = Decimal String To Number(string=w438, default (0L)=w434) -> (number=w429:u16)  [unwired: 1 in, 1 out]
                  n235 = Decimal String To Number(string=w439, default (0L)=w434) -> (number=w428:u16)  [unwired: 1 in, 1 out]
                  n236 = Decimal String To Number(string=w440, default (0L)=w434) -> (number=w427:u16)  [unwired: 1 in, 1 out]
                  n237 = Bundle By Name(cluster=w451, "PB.Pulse Name"=w435, "PB.Amp Low Limit (uA)"=w432, "PB.Amp Step (uA)"=w431, "PB.Amp Step Index"=w430, "PB.PW Low Limit (uS)"=w429, "PB.PW High Limit (uS)"=w428, "PB.PW Default (uS)"=w427) -> (w450:T10)
                }
                frame 5 {
                  w467 = u16 0  # U16
                  w466 = u8 0  # U8
                  w475 = "="
                  n238 = Pick Line(multi-line string=w476, line index=145) -> (output string=w491:string)  [unwired: 1 in]
                  n239 = Pick Line(multi-line string=w476, line index=146) -> (output string=w489:string)  [unwired: 1 in]
                  n240 = Pick Line(multi-line string=w476, line index=147) -> (output string=w487:string)  [unwired: 1 in]
                  n241 = Pick Line(multi-line string=w476, line index=148) -> (output string=w485:string)  [unwired: 1 in]
                  n242 = Pick Line(multi-line string=w476, line index=149) -> (output string=w481:string)  [unwired: 1 in]
                  n243 = Pick Line(multi-line string=w476, line index=150) -> (output string=w479:string)  [unwired: 1 in]
                  n244 = Pick Line(multi-line string=w476, line index=151) -> (output string=w477:string)  [unwired: 1 in]
                  n245 = Match Pattern(string=w491, regular expression=w475) -> (after substring=w468:string)  [unwired: 1 in, 3 out]
                  n246 = Match Pattern(string=w489, regular expression=w475) -> (after substring=w474:string)  [unwired: 1 in, 3 out]
                  n247 = Match Pattern(string=w487, regular expression=w475) -> (after substring=w469:string)  [unwired: 1 in, 3 out]
                  n248 = Match Pattern(string=w485, regular expression=w475) -> (after substring=w470:string)  [unwired: 1 in, 3 out]
                  n249 = Match Pattern(string=w481, regular expression=w475) -> (after substring=w471:string)  [unwired: 1 in, 3 out]
                  n250 = Match Pattern(string=w479, regular expression=w475) -> (after substring=w472:string)  [unwired: 1 in, 3 out]
                  n251 = Match Pattern(string=w477, regular expression=w475) -> (after substring=w473:string)  [unwired: 1 in, 3 out]
                  n252 = Decimal String To Number(string=w474, default (0L)=w467) -> (number=w465:u16)  [unwired: 1 in, 1 out]
                  n253 = Decimal String To Number(string=w469, default (0L)=w467) -> (number=w464:u16)  [unwired: 1 in, 1 out]
                  n254 = Decimal String To Number(string=w470, default (0L)=w466) -> (number=w463:u8)  [unwired: 1 in, 1 out]
                  n255 = Decimal String To Number(string=w471, default (0L)=w467) -> (number=w462:u16)  [unwired: 1 in, 1 out]
                  n256 = Decimal String To Number(string=w472, default (0L)=w467) -> (number=w461:u16)  [unwired: 1 in, 1 out]
                  n257 = Decimal String To Number(string=w473, default (0L)=w467) -> (number=w460:u16)  [unwired: 1 in, 1 out]
                  n258 = Bundle By Name(cluster=w484, "PC.Pulse Name"=w468, "PC.Amp Low Limit (uA)"=w465, "PC.Amp Step (uA)"=w464, "PC.Amp Step Index"=w463, "PC.PW Low Limit (uS)"=w462, "PC.PW High Limit (uS)"=w461, "PC.PW Default (uS)"=w460) -> (w483:T10)
                }
                frame 6 {
                  w500 = u16 0  # U16
                  w499 = u8 0  # U8
                  w508 = "="
                  n259 = Pick Line(multi-line string=w509, line index=180) -> (output string=w524:string)  [unwired: 1 in]
                  n260 = Pick Line(multi-line string=w509, line index=181) -> (output string=w522:string)  [unwired: 1 in]
                  n261 = Pick Line(multi-line string=w509, line index=182) -> (output string=w520:string)  [unwired: 1 in]
                  n262 = Pick Line(multi-line string=w509, line index=183) -> (output string=w518:string)  [unwired: 1 in]
                  n263 = Pick Line(multi-line string=w509, line index=184) -> (output string=w514:string)  [unwired: 1 in]
                  n264 = Pick Line(multi-line string=w509, line index=185) -> (output string=w512:string)  [unwired: 1 in]
                  n265 = Pick Line(multi-line string=w509, line index=186) -> (output string=w510:string)  [unwired: 1 in]
                  n266 = Match Pattern(string=w524, regular expression=w508) -> (after substring=w501:string)  [unwired: 1 in, 3 out]
                  n267 = Match Pattern(string=w522, regular expression=w508) -> (after substring=w507:string)  [unwired: 1 in, 3 out]
                  n268 = Match Pattern(string=w520, regular expression=w508) -> (after substring=w502:string)  [unwired: 1 in, 3 out]
                  n269 = Match Pattern(string=w518, regular expression=w508) -> (after substring=w503:string)  [unwired: 1 in, 3 out]
                  n270 = Match Pattern(string=w514, regular expression=w508) -> (after substring=w504:string)  [unwired: 1 in, 3 out]
                  n271 = Match Pattern(string=w512, regular expression=w508) -> (after substring=w505:string)  [unwired: 1 in, 3 out]
                  n272 = Match Pattern(string=w510, regular expression=w508) -> (after substring=w506:string)  [unwired: 1 in, 3 out]
                  n273 = Decimal String To Number(string=w507, default (0L)=w500) -> (number=w498:u16)  [unwired: 1 in, 1 out]
                  n274 = Decimal String To Number(string=w502, default (0L)=w500) -> (number=w497:u16)  [unwired: 1 in, 1 out]
                  n275 = Decimal String To Number(string=w503, default (0L)=w499) -> (number=w496:u8)  [unwired: 1 in, 1 out]
                  n276 = Decimal String To Number(string=w504, default (0L)=w500) -> (number=w495:u16)  [unwired: 1 in, 1 out]
                  n277 = Decimal String To Number(string=w505, default (0L)=w500) -> (number=w494:u16)  [unwired: 1 in, 1 out]
                  n278 = Decimal String To Number(string=w506, default (0L)=w500) -> (number=w493:u16)  [unwired: 1 in, 1 out]
                  n279 = Bundle By Name(cluster=w517, "PD.Pulse Name"=w501, "PD.Amp Low Limit (uA)"=w498, "PD.Amp Step (uA)"=w497, "PD.Amp Step Index"=w496, "PD.PW Low Limit (uS)"=w495, "PD.PW High Limit (uS)"=w494, "PD.PW Default (uS)"=w493) -> (w516:T10)
                }
                frame 7 {
                  n280 = for {
                    N: 26 -> [_]
                    tunnel: 82 ("line index") -> [w536]
                    tunnel: w529 -> [w538]
                    tunnel: [w532] -> w526 mode=indexing
                    i -> [w535]
                    n281 = Add(x=w535, y=w536) -> (x+y=w537:i32)
                    n282 = Pick Line(multi-line string=w538, line index=w537) -> (output string=w540:string)  [unwired: 1 in]
                    n283 = Match Pattern(string=w540, regular expression="=") -> (after substring=w534:string)  [unwired: 1 in, 3 out]
                    n284 = Decimal String To Number(string=w534, default (0L)=i8 0 ("default (0 I32)")) -> (number=w532:i8)  [unwired: 1 in, 1 out]
                  }
                  n285 = Bundle By Name(cluster=w531, "PA.Amplitudes"=w526) -> (w530:T10)
                }
                frame 8 {
                  n286 = for {
                    N: 26 -> [_]
                    tunnel: 117 ("line index") -> [w551]
                    tunnel: w544 -> [w553]
                    tunnel: [w547] -> w541 mode=indexing
                    i -> [w550]
                    n287 = Add(x=w550, y=w551) -> (x+y=w552:i32)
                    n288 = Pick Line(multi-line string=w553, line index=w552) -> (output string=w555:string)  [unwired: 1 in]
                    n289 = Match Pattern(string=w555, regular expression="=") -> (after substring=w549:string)  [unwired: 1 in, 3 out]
                    n290 = Decimal String To Number(string=w549, default (0L)=i8 0 ("default (0 I32)")) -> (number=w547:i8)  [unwired: 1 in, 1 out]
                  }
                  n291 = Bundle By Name(cluster=w546, "PB.Amplitudes"=w541) -> (w545:T10)
                }
                frame 9 {
                  n292 = for {
                    N: 26 -> [_]
                    tunnel: 152 ("line index") -> [w566]
                    tunnel: w559 -> [w568]
                    tunnel: [w562] -> w556 mode=indexing
                    i -> [w565]
                    n293 = Add(x=w565, y=w566) -> (x+y=w567:i32)
                    n294 = Pick Line(multi-line string=w568, line index=w567) -> (output string=w570:string)  [unwired: 1 in]
                    n295 = Match Pattern(string=w570, regular expression="=") -> (after substring=w564:string)  [unwired: 1 in, 3 out]
                    n296 = Decimal String To Number(string=w564, default (0L)=i8 0 ("default (0 I32)")) -> (number=w562:i8)  [unwired: 1 in, 1 out]
                  }
                  n297 = Bundle By Name(cluster=w561, "PC.Amplitudes"=w556) -> (w560:T10)
                }
                frame 10 {
                  n298 = for {
                    N: 26 -> [_]
                    tunnel: 187 ("line index") -> [w581]
                    tunnel: w574 -> [w583]
                    tunnel: [w577] -> w571 mode=indexing
                    i -> [w580]
                    n299 = Add(x=w580, y=w581) -> (x+y=w582:i32)
                    n300 = Pick Line(multi-line string=w583, line index=w582) -> (output string=w585:string)  [unwired: 1 in]
                    n301 = Match Pattern(string=w585, regular expression="=") -> (after substring=w579:string)  [unwired: 1 in, 3 out]
                    n302 = Decimal String To Number(string=w579, default (0L)=i8 0 ("default (0 I32)")) -> (number=w577:i8)  [unwired: 1 in, 1 out]
                  }
                  n303 = Bundle By Name(cluster=w576, "PD.Amplitudes"=w571) -> (w575:T10)
                }
              }
            }
            n304 = local write "PatStim"(w315) -> ()
          }
        }
      }
      frame "Top of Loop" {
        # "Force status update every 1s"
        n305 = local read "Get VBAT Cont"() -> (w589:bool)
        n306 = Tick Count (ms)() -> (millisecond timer value=w598:u32)
        n307 = Select(t=u32 2000 ("y"), s=w589, f=u32 500 ("y")) -> (s? t:f=w586:u32)
        n308 = Add(x="Tick Count", y=w586) -> (x+y=w596:u32)
        n309 = Greater?(x=w598, y=w596) -> (0:w595:bool)
        n310 = Select(t=string[] ["Get Status"], s=w595, f=w600) -> (s? t:f=w601:string[])
        n311 = for {
          N: 25 -> [_]
          shift-right: [w606] -> w593
          shift-left: w601 -> [w607]
          i -> [w608]
          n312 = case shown="24" w608 {
            tunnel: w607 -> [w612 w623 w634 w645 w655 w663 w671 w679 w687 w695 w703 w711 w719 w727 w735 w743 w751 w759 w767 w775 w783 w791 w799 w807 w815]
            tunnel: [w609 w620 w631 w642 w654 w662 w670 w678 w686 w694 w702 w710 w718 w726 w734 w742 w750 w758 w766 w774 w782 w790 w798 w806 w814] -> w606
            frame 0, Default {
              # "Update CCA"
              n313 = local read "Base Station RF Control"() -> (w610:T2)
              n314 = Unbundle By Name(w610) -> ("Update CCA"=w611:bool)
              n315 = case shown="True" w611 {
                tunnel: w612 -> [w613 w616]
                tunnel: w610 -> [_ w618]
                tunnel: [w613 w615] -> w609
                frame False {
                }
                frame True {
                  n316 = Bundle By Name(cluster=w618, "Update CCA"=FALSE ("CCA Mode")) -> (w619:T2)
                  n317 = local write "Base Station RF Control"(w619) -> ()
                  n318 = Build Array (concatenate)(w616, string[] ["Get CCA", "Get Status"]) -> (w615:string[])
                }
              }
            }
            frame 1 {
              # "Update CCA"
              n319 = local read "Search for Device"() -> (w621:T3)
              n320 = Unbundle By Name(w621) -> ("Search for Device"=w622:bool)
              n321 = case shown="True" w622 {
                tunnel: w623 -> [w624 w627]
                tunnel: w621 -> [_ w629]
                tunnel: [w624 w626] -> w620
                frame False {
                }
                frame True {
                  n322 = Bundle By Name(cluster=w629, "Search for Device"=FALSE ("CCA Mode")) -> (w630:T3)
                  n323 = local write "Search for Device"(w630) -> ()
                  n324 = Build Array (concatenate)(w627, string[] ["Search for Device", "Get Status"]) -> (w626:string[])
                }
              }
            }
            frame 2 {
              # "Update CCA"
              n325 = local read "Session Control"() -> (w632:T4)
              n326 = Unbundle By Name(w632) -> ("Open Session"=w633:bool)
              n327 = case shown="True" w633 {
                tunnel: w634 -> [w635 w638]
                tunnel: w632 -> [_ w640]
                tunnel: [w635 w637] -> w631
                frame False {
                }
                frame True {
                  n328 = Bundle By Name(cluster=w640, "Open Session"=FALSE ("CCA Mode")) -> (w641:T4)
                  n329 = local write "Session Control"(w641) -> ()
                  n330 = Build Array (concatenate)(w638, string[] ["Open Session", "Get Status"]) -> (w637:string[])
                }
              }
            }
            frame 3 {
              # "Update CCA"
              n331 = local read "Session Control"() -> (w643:T4)
              n332 = Unbundle By Name(w643) -> ("Close Session"=w644:bool)
              n333 = case shown="True" w644 {
                tunnel: w645 -> [w646 w649]
                tunnel: w643 -> [_ w651]
                tunnel: [w646 w648] -> w642
                frame False {
                }
                frame True {
                  n334 = Bundle By Name(cluster=w651, "Close Session"=FALSE ("CCA Mode")) -> (w652:T4)
                  n335 = local write "Session Control"(w652) -> ()
                  n336 = Build Array (concatenate)(w649, string[] ["Close Session", "Get Status"]) -> (w648:string[])
                }
              }
            }
            frame 4 {
              # "Update CCA"
              n337 = case shown="True" "Telem Driver" {
                tunnel: w655 -> [w656 w660]
                tunnel: [w656 w659] -> w654
                frame False {
                }
                frame True {
                  n338 = local write "Telem Driver"(FALSE ("CCA Mode")) -> ()
                  n339 = Build Array (concatenate)(w660, string[] ["Telem Driver", "Get Status"]) -> (w659:string[])
                }
              }
            }
            frame 5 {
              # "Update CCA"
              n340 = case shown="True" "LoadPatProgFromDevice" {
                tunnel: w663 -> [w664 w668]
                tunnel: [w664 w667] -> w662
                frame False {
                }
                frame True {
                  n341 = local write "LoadPatProgFromDevice"(FALSE ("CCA Mode")) -> ()
                  n342 = Build Array (concatenate)(w668, string[] ["Uplink Patient Program", "Get Status"]) -> (w667:string[])
                }
              }
            }
            frame 6 {
              # "Update CCA"
              n343 = case shown="True" "Query Error" {
                tunnel: w671 -> [w672 w676]
                tunnel: [w672 w675] -> w670
                frame False {
                }
                frame True {
                  n344 = local write "Query Error"(FALSE ("CCA Mode")) -> ()
                  n345 = Build Array (concatenate)(w676, string[] ["Get BS Error", "Get Status"]) -> (w675:string[])
                }
              }
            }
            frame 7 {
              # "Update CCA"
              n346 = case shown="True" "UpdatePatProgString" {
                tunnel: w679 -> [w680 w684]
                tunnel: [w680 w683] -> w678
                frame False {
                }
                frame True {
                  n347 = local write "UpdatePatProgString"(FALSE ("CCA Mode")) -> ()
                  n348 = Build Array (concatenate)(w684, string[] ["Build Pat Prog String", "Get Status"]) -> (w683:string[])
                }
              }
            }
            frame 8 {
              # "Update CCA"
              n349 = case shown="True" "SendPatProgToDevice" {
                tunnel: w687 -> [w688 w692]
                tunnel: [w688 w691] -> w686
                frame False {
                }
                frame True {
                  n350 = local write "SendPatProgToDevice"(FALSE ("CCA Mode")) -> ()
                  n351 = Build Array (concatenate)(w692, string[] ["Downlink Patient Program", "Get Status"]) -> (w691:string[])
                }
              }
            }
            frame 9 {
              # "Update CCA"
              n352 = case shown="True" "SetPatProgActive" {
                tunnel: w695 -> [w696 w700]
                tunnel: [w696 w699] -> w694
                frame False {
                }
                frame True {
                  n353 = local write "SetPatProgActive"(FALSE ("CCA Mode")) -> ()
                  n354 = Build Array (concatenate)(w700, string[] ["Set Program Active", "Get Status"]) -> (w699:string[])
                }
              }
            }
            frame 10 {
              # "Update CCA"
              n355 = case shown="True" "StartStimulation" {
                tunnel: w703 -> [w704 w708]
                tunnel: [w704 w707] -> w702
                frame False {
                }
                frame True {
                  n356 = local write "StartStimulation"(FALSE ("CCA Mode")) -> ()
                  n357 = Build Array (concatenate)(w708, string[] ["Start Patient Stim", "Get Status"]) -> (w707:string[])
                }
              }
            }
            frame 11 {
              # "Update CCA"
              n358 = case shown="True" "StopStimulation" {
                tunnel: w711 -> [w712 w716]
                tunnel: [w712 w715] -> w710
                frame False {
                }
                frame True {
                  n359 = local write "StopStimulation"(FALSE ("CCA Mode")) -> ()
                  n360 = Build Array (concatenate)(w716, string[] ["Stop Stimulation", "Get Status"]) -> (w715:string[])
                }
              }
            }
            frame 12 {
              # "Update CCA"
              n361 = case shown="True" "ProgAmpUp" {
                tunnel: w719 -> [w720 w724]
                tunnel: [w720 w723] -> w718
                frame False {
                }
                frame True {
                  n362 = local write "ProgAmpUp"(FALSE ("CCA Mode")) -> ()
                  n363 = Build Array (concatenate)(w724, string[] ["Increment Program Ampl", "Get Status"]) -> (w723:string[])
                }
              }
            }
            frame 13 {
              # "Update CCA"
              n364 = case shown="True" "ProgAmpDn" {
                tunnel: w727 -> [w728 w732]
                tunnel: [w728 w731] -> w726
                frame False {
                }
                frame True {
                  n365 = local write "ProgAmpDn"(FALSE ("CCA Mode")) -> ()
                  n366 = Build Array (concatenate)(w732, string[] ["Decrement Program Ampl", "Get Status"]) -> (w731:string[])
                }
              }
            }
            frame 14 {
              # "Update CCA"
              n367 = case shown="True" "FreqUp" {
                tunnel: w735 -> [w736 w740]
                tunnel: [w736 w739] -> w734
                frame False {
                }
                frame True {
                  n368 = local write "FreqUp"(FALSE ("CCA Mode")) -> ()
                  n369 = Build Array (concatenate)(w740, string[] ["Increment Program Freq", "Get Status"]) -> (w739:string[])
                }
              }
            }
            frame 15 {
              # "Update CCA"
              n370 = case shown="True" "FreqDn" {
                tunnel: w743 -> [w744 w748]
                tunnel: [w744 w747] -> w742
                frame False {
                }
                frame True {
                  n371 = local write "FreqDn"(FALSE ("CCA Mode")) -> ()
                  n372 = Build Array (concatenate)(w748, string[] ["Decrement Program Freq", "Get Status"]) -> (w747:string[])
                }
              }
            }
            frame 16 {
              # "Update CCA"
              n373 = case shown="True" "Get Attenuator" {
                tunnel: w751 -> [w752 w756]
                tunnel: [w752 w755] -> w750
                frame False {
                }
                frame True {
                  n374 = local write "Get Attenuator"(FALSE ("CCA Mode")) -> ()
                  n375 = Build Array (concatenate)(w756, string[] ["Get Attenuator", "Get Status"]) -> (w755:string[])
                }
              }
            }
            frame 17 {
              # "Update CCA"
              n376 = case shown="True" "Set Attenuator" {
                tunnel: w759 -> [w760 w764]
                tunnel: [w760 w763] -> w758
                frame False {
                }
                frame True {
                  n377 = local write "Set Attenuator"(FALSE ("CCA Mode")) -> ()
                  n378 = Build Array (concatenate)(w764, string[] ["Set Attenuator", "Get Status"]) -> (w763:string[])
                }
              }
            }
            frame 18 {
              # "Update CCA"
              n379 = case shown="True" "Do Calibration" {
                tunnel: w767 -> [w768 w772]
                tunnel: [w768 w771] -> w766
                frame False {
                }
                frame True {
                  n380 = local write "Do Calibration"(FALSE ("CCA Mode")) -> ()
                  n381 = Build Array (concatenate)(w772, string[] ["Run Calibration", "Get Status"]) -> (w771:string[])
                }
              }
            }
            frame 19 {
              # "Update CCA"
              n382 = case shown="True" "Get Register" {
                tunnel: w775 -> [w776 w780]
                tunnel: [w776 w779] -> w774
                frame False {
                }
                frame True {
                  n383 = local write "Get Register"(FALSE ("CCA Mode")) -> ()
                  n384 = Build Array (concatenate)(w780, string[] ["Get Register", "Get Status"]) -> (w779:string[])
                }
              }
            }
            frame 20 {
              # "Update CCA"
              n385 = case shown="True" "Set Register" {
                tunnel: w783 -> [w784 w788]
                tunnel: [w784 w787] -> w782
                frame False {
                }
                frame True {
                  n386 = local write "Set Register"(FALSE ("CCA Mode")) -> ()
                  n387 = Build Array (concatenate)(w788, string[] ["Set Register", "Get Status"]) -> (w787:string[])
                }
              }
            }
            frame 21 {
              # "Update CCA"
              n388 = case shown="True" "LoadPatProgFromFile" {
                tunnel: w791 -> [w792 w796]
                tunnel: [w792 w795] -> w790
                frame False {
                }
                frame True {
                  n389 = local write "LoadPatProgFromFile"(FALSE ("CCA Mode")) -> ()
                  n390 = Build Array (concatenate)(w796, string[] ["Load Pat Program", "Get Status"]) -> (w795:string[])
                }
              }
            }
            frame 22 {
              # "Update CCA"
              n391 = case shown="True" "SavePatProgToFile" {
                tunnel: w799 -> [w800 w804]
                tunnel: [w800 w803] -> w798
                frame False {
                }
                frame True {
                  n392 = local write "SavePatProgToFile"(FALSE ("CCA Mode")) -> ()
                  n393 = Build Array (concatenate)(w804, string[] ["Save Pat Program", "Get Status"]) -> (w803:string[])
                }
              }
            }
            frame 23 {
              # "Update CCA"
              n394 = case shown="True" "Dongle Reset" {
                tunnel: w807 -> [w808 w812]
                tunnel: [w808 w811] -> w806
                frame False {
                }
                frame True {
                  n395 = local write "Dongle Reset"(FALSE ("CCA Mode")) -> ()
                  n396 = Build Array (concatenate)(w812, string[] ["Reset Dongle", "Get Status"]) -> (w811:string[])
                }
              }
            }
            frame 24 {
              # "Update CCA"
              n397 = case shown="True" "ZL Mass Read" {
                tunnel: w815 -> [w816 w820]
                tunnel: [w816 w819] -> w814
                frame False {
                }
                frame True {
                  n398 = local write "ZL Mass Read"(FALSE ("CCA Mode")) -> ()
                  n399 = Build Array (concatenate)(w820, string[] ["ZL Register Mass Read", "Get Status"]) -> (w819:string[])
                }
              }
            }
          }
        }
        n400 = Wait (ms)(milliseconds to wait=u32 100) -> ()  [unwired: 1 out]
        n401 = Array Size(array=w593) -> (size(s)=w592:i32)
        n402 = Greater?(x=w592, y=1) -> (0:w590:bool)
        n403 = property on="Busy Flag" class="Str"("Visible"=w590) -> ()  [unwired: 2 in, 2 out]
      }
      frame "Get Status" {
        n404 = Tick Count (ms)() -> (millisecond timer value=w833:u32)
        n405 = flat-sequence {
          tunnel: w832 -> [w861]
          tunnel: [w861] -> w831
          frame #0 {
            n406 = Wait (ms)(milliseconds to wait=u32 20) -> ()  [unwired: 1 out]
          }
        }
        n407 = property on="Busy Flag" class="Str"("Visible"=FALSE) -> ()  [unwired: 2 in, 2 out]
        n408 = local write "Tick Count"(w833) -> ()
        n409 = call "MICSD Status.vi"("VISA Resource Name"=w835, "error in (no error)"=w831) -> ("Data Status"=→"Data Status":T7, "dup VISA Resource Name"=w821:refnum<visa-resource-name>, "Status Flags"=w838:T8, "Link Status"=→"Link Status":T5, "Link Quality"=→"Link Quality":T6, "error out"=w830:errorcluster)  [unwired: 7 in, 1 out]
        "Status Flags" <- w838
        n410 = Unbundle By Name(w838) -> ("ERROR_OCCURRED"=→"ERROR":bool, "IDLE"=→"IDLE":bool, "IN_SESSION"=w828:bool)
        "SESSION" <- w828
        n411 = flat-sequence {
          tunnel: w830 -> [w859]
          tunnel: [w859] -> w823
          frame #0 {
            n412 = Wait (ms)(milliseconds to wait=u32 20) -> ()  [unwired: 1 out]
          }
        }
        n413 = Or(x="Get VBAT Cont", y="Get VBAT Single") -> (x .or. y?=w825:bool)
        n414 = And(x=w828, y=w825) -> (x .and. y?=w824:bool)
        n415 = case shown="True" w824 {
          tunnel: w823 -> [w844 w849]
          tunnel: [w844 w857] -> w822
          tunnel: w821 -> [_ w847]
          frame False {
            n416 = local write "Get VBAT Cont"(FALSE ("Get VBAT Cont")) -> ()
          }
          frame True {
            n417 = call "MICSD Telem Driver.vi"("VISA Resource Name"=w847, "Command"=Typedef_Command_List."Charging Control", "error in (no error)"=w849) -> ("Data"=→"Charging Status":string, "error out"=w848:errorcluster)  [unwired: 10 in, 5 out]
            n418 = call "MICSD Telem Driver.vi"("VISA Resource Name"=w847, "Command"=Typedef_Command_List."Get VBAT", "error in (no error)"=w848) -> ("Data"=w855:string, "error out"=w857:errorcluster)  [unwired: 10 in, 5 out]
            n419 = Match Pattern(string=w855, regular expression="=") -> (after substring=w853:string)  [unwired: 1 in, 3 out]
            n420 = Decimal String To Number(string=w853) -> (number=w851:i32)  [unwired: 2 in, 1 out]
            "ADC Counts" <- w851
            n421 = Multiply(x=w851, y=0.001221001) -> (x*y=→"VBAT (Volts)":dbl)
          }
        }
      }
      frame "Build Pat Prog String" {
        n422 = local read "PatStim"() -> (w865:T10)
        n423 = for {
          N: 5 -> [_]
          tunnel: w865 -> [w872]
          shift-right: [w871] -> w864
          shift-left: "" -> [w870]
          i -> [w873]
          n424 = case shown="0, Default" w873 {
            tunnel: w872 -> [w910 w921 w943 w965 w987]
            tunnel: [w880 w924 w946 w968 w990] -> w871
            tunnel: w870 -> [w874 w923 w945 w967 w989]
            frame 0, Default {
              n425 = Unbundle By Name(w910) -> ("Program Number"=w908:u8, "Program Defined"=w877:bool, "Program Disabled"=w878:bool, "Program Name"=w907:string, "Allowed Freq Indexes"=w906:u8[], "Default Freq Index"=w896:u8, "PA.Defined"=w895:bool, "PB.Defined"=w894:bool, "PC.Defined"=w893:bool, "PD.Defined"=w892:bool)
              n426 = local write "Patient Program String"(w874) -> ()
              n427 = Boolean To (0,1)(Boolean=w877) -> (0, 1=w876:i16)
              n428 = Boolean To (0,1)(Boolean=w878) -> (0, 1=w875:i16)
              n429 = Array To Cluster(array=w906) -> (cluster=w905:T18)
              n430 = Boolean To (0,1)(Boolean=w895) -> (0, 1=w881:i16)
              n431 = Boolean To (0,1)(Boolean=w894) -> (0, 1=w889:i16)
              n432 = Boolean To (0,1)(Boolean=w893) -> (0, 1=w890:i16)
              n433 = Boolean To (0,1)(Boolean=w892) -> (0, 1=w891:i16)
              n434 = Logical Shift(y=i8 1, x=w889) -> (x << y=w882:i16)
              n435 = Logical Shift(y=i8 2, x=w890) -> (x << y=w883:i16)
              n436 = Logical Shift(y=i8 3, x=w891) -> (x << y=w884:i16)
              n437 = Compound Arithmetic op=ADD(w881, w882, w883, w884) -> (w885:i16)
              n438 = To Unsigned Byte Integer(number=w885) -> (unsigned 8bit integer=w879:u8)
              n439 = Unbundle(w905) -> ("Allowed Freq Indexes[0]"=w904:u8, "Allowed Freq Indexes[1]"=w903:u8, "Allowed Freq Indexes[2]"=w902:u8, "Allowed Freq Indexes[3]"=w901:u8, "Allowed Freq Indexes[4]"=w900:u8, "Allowed Freq Indexes[5]"=w899:u8, "Allowed Freq Indexes[6]"=w898:u8, "Allowed Freq Indexes[7]"=w897:u8)
              n440 = Format Into String(format string="ProgramNumber=%d\r\nProgramDefined=%d\r\nProgramDisabled=%d\r\nProgramName=%s\r\nAllowedFrequencies[0]=0x%02x\r\nAllowedFrequencies[1]=0x%02x\r\nAllowedFrequencies[2]=0x%02x\r\nAllowedFrequencies[3]=0x%02x\r\nAllowedFrequencies[4]=0x%02x\r\nAllowedFrequencies[5]=0x%02x\r\nAllowedFrequencies[6]=0x%02x\r\nAllowedFrequencies[7]=0x%02x\r\nProgramFrequencyIndex=%d\r\nDefinedPulseMap=0x%02x\r\n", w908, w876, w875, w907, w904, w903, w902, w901, w900, w899, w898, w897, w896, w879) -> (resulting string=w880:string)  [unwired: 2 in, 1 out]
            }
            frame 1 {
              n441 = Unbundle By Name(w921) -> ("PA.Pulse Name"=w920:string, "PA.Amp Low Limit (uA)"=w919:u16, "PA.Amp Step (uA)"=w918:u16, "PA.Amp Step Index"=w917:u16, "PA.PW Low Limit (uS)"=w916:u16, "PA.PW High Limit (uS)"=w915:u16, "PA.PW Default (uS)"=w914:u16, "PA.Amplitudes"=w913:i8[])
              n442 = for {
                tunnel: w913 -> [w932] mode=indexing
                shift-right: [w930] -> w912
                shift-left: "" -> [w931]
                i -> [w928]
                n443 = To Byte Integer(number=w932) -> (8bit integer=w926:i8)
                n444 = Increment(x=w928) -> (x+1=w927:i32)
                n445 = Format Into String(format string="ElectrodeAmpPercentPA[CH%02d]=%d\\r\\n", initial string=w931, w927, w926) -> (resulting string=w930:string)  [unwired: 1 in, 1 out]
              }
              n446 = Format Into String(format string="PulseNamePA=%s\r\nAmplitudeLowLimitPA=%d\r\nAmplitudeStepPA=%d\r\nAmplitudeStepIndexPA=%d\r\nPulseWidthLowLimitPA=%d\r\nPulseWidthHighLimitPA=%d\r\nPulseWidthPA=%d\r\n%s", w920, w919, w918, w917, w916, w915, w914, w912) -> (resulting string=w922:string)  [unwired: 2 in, 1 out]
              n447 = Concatenate Strings(w923, w922) -> (w924:string)
            }
            frame 2 {
              n448 = Unbundle By Name(w943) -> ("PB.Pulse Name"=w942:string, "PB.Amp Low Limit (uA)"=w941:u16, "PB.Amp Step (uA)"=w940:u16, "PB.Amp Step Index"=w939:u16, "PB.PW Low Limit (uS)"=w938:u16, "PB.PW High Limit (uS)"=w937:u16, "PB.PW Default (uS)"=w936:u16, "PB.Amplitudes"=w935:i8[])
              n449 = for {
                tunnel: w935 -> [w954] mode=indexing
                shift-right: [w952] -> w934
                shift-left: "" -> [w953]
                i -> [w950]
                n450 = To Byte Integer(number=w954) -> (8bit integer=w948:i8)
                n451 = Increment(x=w950) -> (x+1=w949:i32)
                n452 = Format Into String(format string="ElectrodeAmpPercentPB[CH%02d]=%d\\r\\n", initial string=w953, w949, w948) -> (resulting string=w952:string)  [unwired: 1 in, 1 out]
              }
              n453 = Format Into String(format string="PulseNamePB=%s\r\nAmplitudeLowLimitPB=%d\r\nAmplitudeStepPB=%d\r\nAmplitudeStepIndexPB=%d\r\nPulseWidthLowLimitPB=%d\r\nPulseWidthHighLimitPB=%d\r\nPulseWidthPB=%d\r\n%s", w942, w941, w940, w939, w938, w937, w936, w934) -> (resulting string=w944:string)  [unwired: 2 in, 1 out]
              n454 = Concatenate Strings(w945, w944) -> (w946:string)
            }
            frame 3 {
              n455 = Unbundle By Name(w965) -> ("PC.Pulse Name"=w964:string, "PC.Amp Low Limit (uA)"=w963:u16, "PC.Amp Step (uA)"=w962:u16, "PC.Amp Step Index"=w961:u16, "PC.PW Low Limit (uS)"=w960:u16, "PC.PW High Limit (uS)"=w959:u16, "PC.PW Default (uS)"=w958:u16, "PC.Amplitudes"=w957:i8[])
              n456 = for {
                tunnel: w957 -> [w976] mode=indexing
                shift-right: [w974] -> w956
                shift-left: "" -> [w975]
                i -> [w972]
                n457 = To Byte Integer(number=w976) -> (8bit integer=w970:i8)
                n458 = Increment(x=w972) -> (x+1=w971:i32)
                n459 = Format Into String(format string="ElectrodeAmpPercentPC[CH%02d]=%d\\r\\n", initial string=w975, w971, w970) -> (resulting string=w974:string)  [unwired: 1 in, 1 out]
              }
              n460 = Format Into String(format string="PulseNamePC=%s\r\nAmplitudeLowLimitPC=%d\r\nAmplitudeStepPC=%d\r\nAmplitudeStepIndexPC=%d\r\nPulseWidthLowLimitPC=%d\r\nPulseWidthHighLimitPC=%d\r\nPulseWidthPC=%d\r\n%s", w964, w963, w962, w961, w960, w959, w958, w956) -> (resulting string=w966:string)  [unwired: 2 in, 1 out]
              n461 = Concatenate Strings(w967, w966) -> (w968:string)
            }
            frame 4 {
              n462 = Unbundle By Name(w987) -> ("PD.Pulse Name"=w986:string, "PD.Amp Low Limit (uA)"=w985:u16, "PD.Amp Step (uA)"=w984:u16, "PD.Amp Step Index"=w983:u16, "PD.PW Low Limit (uS)"=w982:u16, "PD.PW High Limit (uS)"=w981:u16, "PD.PW High Limit (uS)"=w980:u16, "PD.Amplitudes"=w979:i8[])
              n463 = for {
                tunnel: w979 -> [w998] mode=indexing
                shift-right: [w996] -> w978
                shift-left: "" -> [w997]
                i -> [w994]
                n464 = To Byte Integer(number=w998) -> (8bit integer=w992:i8)
                n465 = Increment(x=w994) -> (x+1=w993:i32)
                n466 = Format Into String(format string="ElectrodeAmpPercentPD[CH%02d]=%d\\r\\n", initial string=w997, w993, w992) -> (resulting string=w996:string)  [unwired: 1 in, 1 out]
              }
              n467 = Format Into String(format string="PulseNamePD=%s\r\nAmplitudeLowLimitPD=%d\r\nAmplitudeStepPD=%d\r\nAmplitudeStepIndexPD=%d\r\nPulseWidthLowLimitPD=%d\r\nPulseWidthHighLimitPD=%d\r\nPulseWidthPD=%d\r\n%s", w986, w985, w984, w983, w982, w981, w980, w978) -> (resulting string=w988:string)  [unwired: 2 in, 1 out]
              n468 = Concatenate Strings(w989, w988) -> (w990:string)
            }
          }
        }
        n469 = local write "Patient Program String"(w864) -> ()
      }
      frame "Downlink Patient Program" {
        n470 = call "MICSD Telem Driver.vi"("VISA Resource Name"=w999, "Command"=Typedef_Command_List."Set Program Definition", "Parameters"="Patient Program String", "error in (no error)"=w1007) -> ("Response Token"=w1004:string, "Response Code"=w1003:string, "error out"=w1006:errorcluster)  [unwired: 9 in, 4 out]
        n471 = Concatenate Strings(w1004, " - ", w1003) -> (w1002:string)
        n472 = local write "Response"(w1002) -> ()
      }
      frame "Set Program Active" {
        n473 = local read "PatStim"() -> (w1011:T10)
        n474 = Unbundle By Name(w1011) -> ("Program Number"=w1010:u8)
        n475 = Format Into String(format string="Program=%d", w1010) -> (resulting string=w1013:string)  [unwired: 2 in, 1 out]
        n476 = call "MICSD Telem Driver.vi"("VISA Resource Name"=w1014, "Command"=Typedef_Command_List."Select Program", "Parameters"=w1013, "error in (no error)"=w1021) -> ("Response Token"=w1018:string, "Response Code"=w1017:string, "error out"=w1020:errorcluster)  [unwired: 9 in, 4 out]
        n477 = Concatenate Strings(w1018, " - ", w1017) -> (w1016:string)
        n478 = local write "Response"(w1016) -> ()
      }
      frame "Start Patient Stim" {
        n479 = call "MICSD Telem Driver.vi"("VISA Resource Name"=w1025, "Command"=Typedef_Command_List."xPG Stimulation", "Parameters"="StimState=1" ("format string"), "error in (no error)"=w1032) -> ("Response Token"=w1029:string, "Response Code"=w1028:string, "error out"=w1031:errorcluster)  [unwired: 9 in, 4 out]
        n480 = Concatenate Strings(w1029, " - ", w1028) -> (w1027:string)
        n481 = local write "Response"(w1027) -> ()
      }
      frame "Stop Stimulation" {
        n482 = call "MICSD Telem Driver.vi"("VISA Resource Name"=w1036, "Command"=Typedef_Command_List."xPG Stimulation", "Parameters"="StimState=0" ("format string"), "error in (no error)"=w1043) -> ("Response Token"=w1040:string, "Response Code"=w1039:string, "error out"=w1042:errorcluster)  [unwired: 9 in, 4 out]
        n483 = Concatenate Strings(w1040, " - ", w1039) -> (w1038:string)
        n484 = local write "Response"(w1038) -> ()
      }
      frame "Get BS Error" {
        n485 = call "MICSD Get Info.vi"("error in (no error)"=w1051, "Command"=T14."Get Device Error", "VISA Resource Name"=w1050) -> ("error out"=w1049:errorcluster, "Response"=→"Base Station Errors Query":string, "dup VISA Resource Name"=w1048:refnum<visa-resource-name>)  [unwired: 6 in]
      }
      frame "Save Pat Program" {
        n486 = Open/Create/Replace File(error in=w1055, prompt="Load Patient Program", operation (0:open)=T15."replace or create with confirmation", access (0:read/write)=enum16{"read/write", "read-only", "write-only"}."write-only") -> (refnum out=w1057:refnum<file>, cancelled=w1056:bool, error out=w1058:errorcluster)  [unwired: 2 in]
        n487 = case shown="False" w1056 {
          tunnel: w1058 -> [w1068 _]
          tunnel: w1057 -> [w1067 _]
          frame False {
            n488 = local read "PatStim"() -> (w1064:T10)
            n489 = Write to Binary File(file (use dialog)=w1067, data=w1064, error in=w1068) -> (refnum out=w1065:refnum<file>, error out=w1066:errorcluster)  [unwired: 3 in, 1 out]
            n490 = case shown="No Error" w1066 {
              selector: w1066 -> [w1070 _]
              tunnel: w1065 -> [w1069 _]
              frame No Error {
                n491 = Close File(refnum=w1069, error in=w1070) -> ()  [unwired: 2 out]
              }
              frame Error {
              }
            }
          }
          frame True {
          }
        }
      }
      frame "Load Pat Program" {
        n492 = Open/Create/Replace File(error in=w1075, prompt="Load Patient Program", access (0:read/write)=enum16{"read/write", "read-only", "write-only"}."read-only") -> (refnum out=w1072:refnum<file>, cancelled=w1071:bool, error out=w1073:errorcluster)  [unwired: 3 in]
        n493 = case shown="False" w1071 {
          tunnel: w1073 -> [w1085 _]
          tunnel: w1072 -> [w1084 _]
          frame False {
            n494 = local read "PatStim"() -> (w1083:T10)
            n495 = Read from Binary File(5:w1083, 8:w1085, 11:w1084) -> (0:w1082:errorcluster, 2:w1081:T10, 3:w1080:refnum<file>)  [unwired: 3 in, 1 out]
            n496 = case shown="No Error" w1082 {
              selector: w1082 -> [w1087 _]
              tunnel: w1081 -> [w1088 _]
              tunnel: w1080 -> [w1086 _]
              frame No Error {
                n497 = local write "PatStim"(w1088) -> ()
                n498 = Close File(refnum=w1086, error in=w1087) -> ()  [unwired: 2 out]
              }
              frame Error {
              }
            }
          }
          frame True {
          }
        }
      }
      frame "Set Attenuator" {
        n499 = Multiply(x="Attenuation (dB)", y=4.0) -> (x*y=w1090:dbl)
        n500 = To Unsigned Byte Integer(number=w1090) -> (unsigned 8bit integer=w1089:u8)
        n501 = call "MICSD Set Attenuator.vi"("error in (no error)"=w1096, "Attenuation"=w1089, "VISA Resource Name"=w1095) -> ("error out"=w1094:errorcluster, "dup VISA Resource Name"=w1093:refnum<visa-resource-name>)  [unwired: 7 in]
      }
      frame "Run Calibration" {
        # "* defines to select group 1 cals */\nCAL_WAKEUP_STROBE_OSC     0x01\nCAL_TX_IF_OSC             0x02\nCAL_FM_DETECT_AND_RX_IF   0x04\nCAL_RX_ADC                0x08\nCAL_400_MHZ_TX_102        0x10  \nCAL_400_MHZ_RX_102        0x20\nCAL_400_MHZ_ANT           0x40\nCAL_24_MHZ_CRYSTAL_OSC    0x80\n/* defines to select group 2 cals/\nCAL_2_MHZ_OSC_102         (0x01 << 8) \nCAL_LNA_FREQ_102          (0x02 << 8)"
        n502 = Build Array("CAL_WAKEUP_STROBE_OSC", "CAL_TX_IF_OSC", "CAL_FM_DETECT_AND_RX_IF", "CAL_RX_ADC", "CAL_400_MHZ_TX", "CAL_400_MHZ_RX", "CAL_400_MHZ_ANT", "CAL_24MHZ_CRYSTAL_OSC") -> (w1100:bool[])
        n503 = Boolean Array To Number(Boolean array=w1100) -> (number=w1099:u32)
        n504 = call "MICSD Calibrate.vi"("VISA Resource Name"=w1114, "Execute on Remote?(F)"="Execute on Remote?(F)", "CalSelect1"=w1099, "Channel"="MICS Channel", "error in (no error)"=w1115) -> ("dup VISA Resource Name"=w1113:refnum<visa-resource-name>, "error out"=w1112:errorcluster)  [unwired: 9 in]
        n505 = flat-sequence {
          tunnel: w1112 -> [w1119]
          tunnel: [w1119] -> w1111
          frame #0 {
            n506 = Wait (ms)(milliseconds to wait=u32 300) -> ()  [unwired: 1 out]
          }
        }
      }
      frame "Set Register" {
        n507 = local read "Register"() -> (w1120:u16)
        n508 = Not Equal?(x=w1120, y=u16 1000) -> (x != y?=w1121:bool)
        n509 = case shown="True" w1121 {
          tunnel: w1120 -> [_ w1132]
          frame False {
          }
          frame True {
            n510 = local write "Address"(w1132) -> ()
          }
        }
        n511 = call "MICSD Set Register.vi"("Execute on Remote?(F)"="Use Remote?", "error in (no error)"=w1129, "Data"="Set Data", "Address"="Address", "VISA Resource Name"=w1128) -> ("error out"=w1124:errorcluster, "dup VISA Resource Name"=w1123:refnum<visa-resource-name>)  [unwired: 5 in]
      }
      frame "Get Register" {
        n512 = Not Equal?(x="Register", y=u16 1000) -> (x != y?=w1134:bool)
        n513 = case shown="True" w1134 {
          tunnel: "Register" -> [_ w1145]
          frame False {
          }
          frame True {
            n514 = local write "Address"(w1145) -> ()
          }
        }
        n515 = local read "Use Remote?"() -> (w1137:bool)
        n516 = local read "Address"() -> (w1138:u16)
        n517 = call "MICSD Get Register.vi"("Execute on Remote?(F)"=w1137, "error in (no error)"=w1142, "Address"=w1138, "VISA Resource Name"=w1141) -> ("error out"=w1140:errorcluster, "Data"=→"Get Data" →"Get Data Dec":u8, "dup VISA Resource Name"=w1139:refnum<visa-resource-name>)  [unwired: 5 in]
      }
      frame "ZL Register Mass Read" {
        n518 = local read "Use Remote?"() -> (w1153:bool)
        n519 = for {
          N: 255 -> [_]
          tunnel: w1153 -> [w1163]
          shift-right: [w1164] -> w1154
          shift-left: w1155 -> [w1166]
          shift-right: [w1165] -> w1150
          shift-left: w1156 -> [w1167]
          tunnel: [w1161] -> w1149 mode=indexing
          i -> [w1162]
          n520 = call "MICSD Get Register.vi"("Execute on Remote?(F)"=w1163, "error in (no error)"=w1167, "Address"=w1162, "VISA Resource Name"=w1166) -> ("error out"=w1165:errorcluster, "Data"=w1161:u8, "dup VISA Resource Name"=w1164:refnum<visa-resource-name>)  [unwired: 5 in]
        }
        n521 = call "MICSD Format Hex Table.vi"("Read Data"=w1149) -> ("String"=w1148:string)  [unwired: 4 in]
        n522 = Write to Text File(file (use dialog)="File Path", text=w1148, error in=w1150) -> (refnum out=w1146:refnum<file>, error out=w1147:errorcluster)  [unwired: 1 in, 1 out]
        n523 = case shown="No Error" w1147 {
          selector: w1147 -> [w1160 _]
          tunnel: w1146 -> [w1159 _]
          frame No Error {
            n524 = Close File(refnum=w1159, error in=w1160) -> ()  [unwired: 2 out]
          }
          frame Error {
          }
        }
      }
      frame "Get Attenuator" {
        n525 = call "MICSD Get Attenuator.vi"("error in (no error)"=w1174, "VISA Resource Name"=w1173) -> ("error out"=w1172:errorcluster, "Attenuation"=w1168:u8, "dup VISA Resource Name"=w1171:refnum<visa-resource-name>)  [unwired: 7 in]
        n526 = Divide(x=w1168, y=4.0) -> (x/y=w1169:dbl)
        n527 = local write "Attenuation (dB)"(w1169) -> ()
      }
      frame "Reset Dongle" {
        n528 = call "MICSD Reset.vi"("error in (no error)"=w1179, "VISA Resource Name"=w1180) -> ("error out"=w1177:errorcluster, "dup VISA Resource Name"=w1178:refnum<visa-resource-name>)  [unwired: 8 in]
      }
      frame "Get CCA" {
        n529 = local read "Base Station RF Control"() -> (w1191:T2)
        n530 = Unbundle By Name(w1191) -> ("RSSI Measurement"=w1189:u16, "Use Averaging?"=w1190:bool)
        n531 = call "MICSD Do CCA.vi"("error in (no error)"=w1194, "Use Averaging?"=w1190, "RSSI Mode"=w1189, "VISA Resource Name"=w1193) -> ("error out"=w1192:errorcluster, "CCA Data"=w1184:u16[], "Selected Channel"=w1188:u8, "dup VISA Resource Name"=w1183:refnum<visa-resource-name>)  [unwired: 4 in]
        n532 = Increment(x=w1188) -> (x+1=w1187:u8)
        n533 = Build Array (concatenate)(u16[] [0] ("CCA Data"), w1184) -> (w1185:u16[])
        n534 = Bundle By Name(cluster=w1191, "Manual RF CH:"=w1187, "Base Station CCA Results"=w1185) -> (w1195:T2)
        n535 = local write "Base Station RF Control"(w1195) -> ()
      }
    }
    n536 = Or(x="stop", y=w16) -> (x .or. y?=w17:bool)
    "Error Monitor" <- w18
  }
  "error out" <- w12
  n537 = local read "Search for Device"() -> (w8:T3)
  n538 = local read "Session Control"() -> (w9:T4)
  n539 = Unbundle By Name(w8) -> ()  [unwired: 1 out]
  n540 = Unbundle By Name(w9) -> ()  [unwired: 2 out]
  n541 = VISA Close(VISA resource name=w1) -> ()  [unwired: 1 in, 1 out]
